vi "Stress Control Test.vi"() -> ()   [LabVIEW 2014]
uses:
  support/Instrument Status.ctl
  Spectrometer/Laser.ctl
  Spectrometer/Spectrometer Config.ctl
  Spectrometer/Laser Settings.ctl
  Spectrometer/Filter.ctl
  Spectrometer/Grating Detector Settings.ctl
  Spectrometer/Grating.ctl
  Spectrometer/Detector.ctl
  Spectrometer/Acquisition Settings.ctl
  Switches and Mirrors/SwitchesMirrors Config.ctl
  Switches and Mirrors/SwitchesMirrors Status.ctl
  Camera/Camera Config.ctl
  Camera/Camera Settings.ctl
  StressControl Config.ctl
  StressControl Refnums.ctl
  Parameter Analyzer/Parameter Analyzer Config.ctl
  Parameter Analyzer/Parameter Analyzer Integration Parameters.ctl
  Parameter Analyzer/Parameter Analyzer SMU Sweeping.ctl
  Parameter Analyzer/Parameter Analyzer Sweep Spacing.ctl
  Parameter Analyzer/Parameter Analyzer SMU Range.ctl
  Parameter Analyzer/Parameter Analyzer SMU Sampling.ctl
  Parameter Analyzer/Parameter Analyzer Sampling Parameters.ctl
  Parameter Analyzer/Parameter Analyzer Stop Sampling Conditions.ctl
  Switching Matrix/Switching Matrix Config.ctl
  XYZ Stage/XYZ Config.ctl
  XYZ Stage/XYZ Connection Settings.ctl
  XYZ Stage/XYZ Stage Control.ctl
  XYZ Stage/XYZ Coordinate Control.ctl
  Autofocus/AutoFocus Config.ctl
  Autofocus/ZScan.ctl
  <vilib>/Analysis/Matrix/Datatypes/RealMatrix.ctl
  Measurements/Strain Measurement/Strain Measurement Config.ctl
  Measurements/Plot Data/PlotData Config.ctl
  Measurements/Plot Data/Measurement.ctl
  Measurements/Plot Data/WhichInstrument.ctl
  Parameter Analyzer/Electrical Data.ctl
  Spectrometer/Spectral Data.ctl
  Measurements/Instrument Sequence/Instrument Steps.ctl
  Measurements/Instrument Sequence/Action.ctl
  Measurements/Instrument Sequence/Instrument List.ctl
  support/User Event - Stop/User Event - Stop.lvlib
  support/Message Queue/Message Queue.lvlib
  <vilib>/Analysis/Matrix/NI_Matrix.lvlib
panel:
  out "Instrument Status":T1
  in  "Mechanism Motion":u16(ring) items=["Absolute", "Relative"]
  in  "Apply Stress":bool
  out "Position (°)":dbl format="%.6g"
  in  "Destination (°)":dbl min=-2000000000.0 max=2000000000.0 format="%.6f"
  in  "Stop":bool
  out "Last Operation":string
  in  "Exit":bool
  # "LICENSED MATERIALS – PROPERTY OF IBM\nCopyright IBM Corp. 2016,\nALL RIGHTS RESERVED"
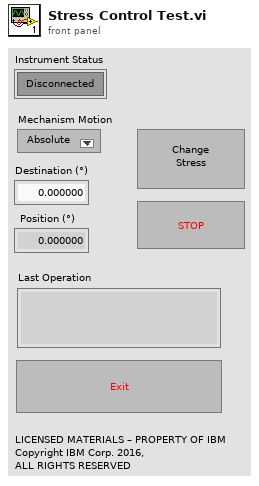
[diagram p1: front panel]
types:
  T1 = typedef "Instrument Status.ctl" = bool
  T2 = typedef "Message Queue.lvlib/All Message Queues.ctl" = cluster{"Message Handler Loop":refnum<queue>, "Parameter Analyzer":refnum<queue>, "Switching Matrix":refnum<queue>, "Stress Control":refnum<queue>, "Optical Spectrometer":refnum<queue>, "Switches & Mirrors":refnum<queue>, "Camera":refnum<queue>, "XYZ Stage":refnum<queue>, "AutoFocus":refnum<queue>, "Optoelectronic":refnum<queue>, "Save Data":refnum<queue>, "Plot Data":refnum<queue>, "Instrument Sequence":refnum<queue>, "Strain Measurement":refnum<queue>}
  T3 = typedef "Notifiers.ctl" = cluster{"Message Handler Loop":T4, "Parameter Analyzer":T5, "Switching Matrix":T6, "Stress Control":T7, "Optical Spectrometer":T8, "Switches & Mirrors":T9, "Camera":T10, "XYZ Stage":T11, "AutoFocus":T12, "Optoelectronic":T13, "Save Data":T14, "Plot Data":T14, "Instrument Sequence":T15, "Strain Measurement":cluster{"Status":refnum<notifier>, "Exit":refnum<notifier>, "Ready":refnum<notifier>}}
  T4 = typedef "Message Handler Loop Notifiers.ctl" = cluster{"Status":refnum<notifier>, "Instrument Data":refnum<notifier>, "Exit":refnum<notifier>, "Ready":refnum<notifier>}
  T5 = typedef "Parameter Analyzer Notifiers.ctl" = cluster{"Status":refnum<notifier>, "Instrument Data":refnum<notifier>, "Measurement":refnum<notifier>, "Exit":refnum<notifier>, "Ready":refnum<notifier>}
  T6 = typedef "Switching Matrix Notifiers.ctl" = cluster{"Status":refnum<notifier>, "Instrument Data":refnum<notifier>, "Measurement":refnum<notifier>, "Exit":refnum<notifier>, "Ready":refnum<notifier>}
  T7 = typedef "StressControl Notifiers.ctl" = cluster{"Status":refnum<notifier>, "Instrument Data":refnum<notifier>, "Measurement":refnum<notifier>, "Exit":refnum<notifier>, "Ready":refnum<notifier>}
  T8 = typedef "Spectrometer Notifiers.ctl" = cluster{"Status":refnum<notifier>, "Instrument Data":refnum<notifier>, "Measurement":refnum<notifier>, "Exit":refnum<notifier>, "Ready":refnum<notifier>}
  T9 = typedef "SwitchesMirrors Notifiers.ctl" = cluster{"Status":refnum<notifier>, "Instrument Data":refnum<notifier>, "Exit":refnum<notifier>, "Ready":refnum<notifier>}
  T10 = typedef "Camera Notifiers.ctl" = cluster{"Status":refnum<notifier>, "Instrument Data":refnum<notifier>, "Measurement":refnum<notifier>, "Exit":refnum<notifier>, "Ready":refnum<notifier>}
  T11 = typedef "XYZ Notifications.ctl" = cluster{"Status":refnum<notifier>, "Instrument Data":refnum<notifier>, "Measurement":refnum<notifier>, "Exit":refnum<notifier>, "Ready":refnum<notifier>}
  T12 = typedef "Autofocus Notifiers.ctl" = cluster{"Status":refnum<notifier>, "Instrument Data":refnum<notifier>, "Measurement":refnum<notifier>, "Exit":refnum<notifier>, "Ready":refnum<notifier>}
  T13 = typedef "Optoelectronic Notifiers.ctl" = cluster{"Status":refnum<notifier>, "Instrument Data":refnum<notifier>, "Measurement":refnum<notifier>, "Exit":refnum<notifier>, "Ready":refnum<notifier>}
  T14 = typedef "SaveData Notifiers.ctl" = cluster{"Status":refnum<notifier>, "Exit":refnum<notifier>, "Ready":refnum<notifier>}
  T15 = typedef "Instrument Sequence Notifiers.ctl" = cluster{"Status":refnum<notifier>, "Instrument Data":refnum<notifier>, "Measurement":refnum<notifier>, "Exit":refnum<notifier>, "Ready":refnum<notifier>}
  T16 = typedef "Configuration.ctl" = cluster{"Parameter Analizer":T17, "Switching Matrix":T25, "Stress Control":T26, "Optical Spectrometer":T27, "Switches & Mirrors":T35, "Camera":T37, "XYZ Stage":T39, "AutoFocus":T43, "Sava Data":T46, "PlotData":T51, "Instrument Sequence":T57, "Strain Measurement":T58}
  T17 = typedef "Parameter Analyzer Config.ctl" = cluster{"Parameter Analyzer VISA Session":refnum<visa-resource-name>, "Sweeping Time Parameters":T18, "Acquisition Mode":enum32{"Sweeping Mode", "Sampling Mode"}, "Status Polling Time (ms)":u32, "Comment":string, "SMU 1 - Sweeping":T19, "SMU 2 - Sweeping":T19, "SMU 3 - Sweeping":T19, "SMU 4 - Sweeping":T19, "Sweep Spacing":T20, "Range":T21, "SMU1 - Sampling":T22, "SMU2 - Sampling":T22, "SMU3 - Sampling":T22, "SMU4 - Sampling":T22, "Sampling Time Parameters":T23, "Stop Condition":T24}
  T18 = typedef "Parameter Analyzer Integration Parameters.ctl" = cluster{"Integration Time":u32, "Short Integration Time (s)":dbl, "Long Integration Time (s)":dbl, "Wait Time Parameter":dbl}
  T19 = typedef "Parameter Analyzer SMU Sweeping.ctl" = cluster{"Start / Offset":dbl, "Stop / Ratio":dbl, "Step \n(linear only)":dbl, "Compliance":dbl, "Power \nCompliance":dbl, "Mode":u32, "Function":i32, "Sweep Mode":bool}
  T20 = typedef "Parameter Analyzer Sweep Spacing.ctl" = u16
  T21 = typedef "Parameter Analyzer SMU Range.ctl" = u16
  T22 = typedef "Parameter Analyzer SMU Sampling.ctl" = cluster{"Source":dbl, "Compliance":dbl, "Mode":u32, "Function":bool}
  T23 = typedef "Parameter Analyzer Sampling Parameters.ctl" = cluster{"Initial Interval (s)":dbl, "Number of Samples":i32, "Total Sampling Time (s)":dbl, "Hold Time (s)":dbl, "Sampling Mode":i32, "Sampling Time":i32}
  T24 = typedef "Parameter Analyzer Stop Sampling Conditions.ctl" = cluster{"Enable Delay (s)":dbl, "Name":string, "Threshold":dbl, "num. of events":i32, "Event":i32, "Stop Condition Enable":bool}
  T25 = typedef "Switching Matrix Config.ctl" = cluster{"Switching Matrix VISA Session":refnum<visa-resource-name>, "Connections":cluster{"Connections":bool[], "Connection Type":enum16{"Disconnected", "Make - Break", "Break - Make"}}[]}
  T26 = typedef "StressControl Config.ctl" = cluster{"Stress Control VISA Session":refnum<visa-resource-name>, "Axis":i32, "Motion":u16, "Destination (°)":dbl, "Speed (°/s)":dbl, "Position (°)":dbl}
  T27 = typedef "Spectrometer Config.ctl" = cluster{"Laser Settings":T28, "Spectrometer Settings":T31, "Acquisition Settings":T34, "Path":path}
  T28 = typedef "Laser Settings.ctl" = cluster{"Laser Wavelength":T29, "Neutral Density Filter":T30}
  T29 = typedef "Laser.ctl" = enum16{"633 nm", "784 nm", "532 nm", "365 nm"}
  T30 = typedef "Filter.ctl" = enum16{"100%", "50%", "25%", "10%", "1%", "0.1%", "0.01%"}
  T31 = typedef "Grating Detector Settings.ctl" = cluster{"Confocal Hole Size (µm)":dbl, "Grating":T32, "Detector":T33}
  T32 = typedef "Grating.ctl" = u16
  T33 = typedef "Detector.ctl" = enum16{"InGaAs Array", "Silicon CCD"}
  T34 = typedef "Acquisition Settings.ctl" = cluster{"Acquisition Mode":enum16{"Single Window", "Multi-Window"}, "Spectal Position (nm)":dbl, "From (nm)":dbl, "To (nm)":dbl, "Integration Time (s)":dbl, "Number of Accumulations":i32, "AutoScanning":bool, "Spike Removal":bool}
  T35 = typedef "SwitchesMirrors Config.ctl" = cluster{"Relay VISA Session":refnum<visa-resource-name>, "Switches":T36, "Delays (ms)":cluster{"Laser":u32, "Video":u32}}
  T36 = typedef "SwitchesMirrors Status.ctl" = cluster{"Laser":bool, "Video":bool}
  T37 = typedef "Camera Config.ctl" = cluster{"Settings":T38}
  T38 = typedef "Camera Settings.ctl" = cluster{"Pixel clock":i32, "Frame rate":dbl, "Exposure time":dbl, "Master Gain":i32, "Red Gain":i32, "Green Gain":i32, "Blue Gain":i32, "Auto Gain":bool, "White-balance":bool, "Color Correction":bool}
  T39 = typedef "XYZ Config.ctl" = cluster{"Connection Settings":T40, "Manual Control":T41, "Coordinate Control":T42}
  T40 = typedef "XYZ Connection Settings.ctl" = cluster{"Tango VISA":refnum<visa-resource-name>, "Baudrate":i32, "Show Protocol?":bool}
  T41 = typedef "XYZ Stage Control.ctl" = cluster{"North":bool, "South":bool, "West":bool, "East":bool, "Up":bool, "Down":bool, "Stop":bool, "XY Step":dbl, "Z step":dbl}
  T42 = typedef "XYZ Coordinate Control.ctl" = cluster{"Motion Mode":enum16{"Absolute", "Relative"}, "Destination [mm]":dbl[]}
  T43 = typedef "AutoFocus Config.ctl" = cluster{"Matching Criteria":cluster{"Minimum Score":sgl, "Color Score Weight":sgl, "Minimum Contrast":i32, "Match Mode":u32, "Match Feature Mode":u32, "Subpixel Accuracy":bool, "Color Sensitivity":u32, "Search Strategy":u32}, "Z Scan Parameters":T44, "Displacement":dbl, "Transformation Matrix":T45}
  T44 = typedef "ZScan.ctl" = cluster{"Z Range":ext, "Resolution":dbl, "Initial Direction":enum16{"Up", "Down"}, "Focus Threshold":dbl, "Ascent Constant":dbl}
  T45 = typedef "NI_Matrix.lvlib/RealMatrix.ctl" = dbl[][]
  T46 = typedef "SaveData Config.ctl" = cluster{"Workspace Info":T47, "Instrument Configuration":T48, "Stress Motor Position":dbl, "Electrical Measurement":cluster{"Sequence":dbl[], "V1":dbl[], "V2":dbl[], "V3":dbl[], "V4":dbl[], "I1":dbl[], "I2":dbl[], "I3":dbl[], "I4":dbl[]}, "Optical Spectrum":T50}
  T47 = typedef "SaveData Workspace Info.ctl" = cluster{"Device Name":string, "Device Info":string, "Path":path}
  T48 = typedef "SaveData Instrument Configuration.ctl" = cluster{"Instrument":T49, "Configuration":string}
  T49 = typedef "Instrument List.ctl" = enum32{"Unknown Instrument", "Switching Matrix", "Parameter Analyzer", "Optical Spectrometer", "Optoelectronic", "Autofocus"}
  T50 = typedef "Spectral Data.ctl" = cluster{"Intensity":dbl[], "Wavelength":dbl[], "Energy":dbl[], "Raman Shift":dbl[], "Detector Temperature":dbl}
  T51 = typedef "PlotData Config.ctl" = cluster{"Sliders":cluster{"Strain Sequence":i32, "Instrument Sequence":i32}, "Measurement":T52, "Instrument Steps":T55, "Strain Points":dbl[]}
  T52 = typedef "Measurement.ctl" = cluster{"Which Instrument?":T53, "Electrical Measurement":T54, "Measurement Mode":enum16{"Sweeping Mode", "Sampling Mode"}, "Optical Spectrum":T50}
  T53 = typedef "WhichInstrument.ctl" = enum16{"No Plot", "Spectrometer", "Parameter Analyzer", "Optoelectronic"}
  T54 = typedef "Electrical Data.ctl" = cluster{"Sequence":dbl[], "V1":dbl[], "V2":dbl[], "V3":dbl[], "V4":dbl[], "I1":dbl[], "I2":dbl[], "I3":dbl[], "I4":dbl[]}
  T55 = typedef "Instrument Steps.ctl" = cluster{"Action":T56, "Configuration":variant, "Instrument":T49, "Status":enum8{"False", "True", "Mixed"}}[]
  T56 = typedef "Action.ctl" = enum32{"Configure", "Measure"}
  T57 = typedef "Instrument Sequence Config.ctl" = cluster{"Caller VI":enum16{"User", "Stress Measurement VI"}}
  T58 = typedef "Strain Measurement Config.ctl" = cluster{"Stress Sequence ":cluster{"Max Motor Position":ext, "# Intermediate Points":u32, "Initial Direction":enum16{"Tension", "Compression"}}, "Track?":bool}
  T59 = typedef "StressControl Refnums.ctl" = cluster{"Instrument Status":refnum<vi>, "Position":refnum<vi>, "Mecahnism Motion":refnum<vi>, "Destination":refnum<vi>, "Apply Stress":refnum<vi>, "Stop":refnum<vi>, "Stress Control VISA":refnum<vi>}
  T60 = cluster{"SMU 1 - Sweeping":cluster{"Start / Offset":dbl, "Stop / Ratio":dbl, "Step (linear only)":dbl, "Compliance":dbl, "Power Compliance":dbl, "Mode":u32, "Function":i32, "Sweep Mode":bool}, "SMU 2 - Sweeping":cluster{"Start / Offset":dbl, "Stop / Ratio":dbl, "Step (linear only)":dbl, "Compliance":dbl, "Power Compliance":dbl, "Mode":u32, "Function":i32, "Sweep Mode":bool}, "SMU 3 - Sweeping":cluster{"Start / Offset":dbl, "Stop / Ratio":dbl, "Step (linear only)":dbl, "Compliance":dbl, "Power Compliance":dbl, "Mode":u32, "Function":i32, "Sweep Mode":bool}, "SMU 4 - Sweeping":cluster{"Start / Offset":dbl, "Stop / Ratio":dbl, "Step (linear only)":dbl, "Compliance":dbl, "Power Compliance":dbl, "Mode":u32, "Function":i32, "Sweep Mode":bool}, "Sweep Spacing":u16, "Range":u16}
  T61 = cluster{"SMU1 - Sampling":cluster{"Source":dbl, "Compliance":dbl, "Mode":u32, "Function":bool}, "SMU2 - Sampling":cluster{"Source":dbl, "Compliance":dbl, "Mode":u32, "Function":bool}, "SMU3 - Sampling":cluster{"Source":dbl, "Compliance":dbl, "Mode":u32, "Function":bool}, "SMU4 - Sampling":cluster{"Source":dbl, "Compliance":dbl, "Mode":u32, "Function":bool}, "Sampling Parameters":cluster{"Initial Interval (s)":dbl, "Number of Samples":i32, "Total Sampling Time (s)":dbl, "Hold Time (s)":dbl, "Sampling Mode":i32, "Sampling Time":i32}, "Stop Condition":cluster{"Enable Delay (s)":dbl, "Name":string, "Threshold":dbl, "num. of events":i32, "Event":i32, "Stop Condition Enable":bool}}
  T62 = cluster{"PlotData - Instrument Sequence":i32, "PlotData - Strain Sequence":i32}
  T63 = cluster{"Start / Offset":dbl, "Stop / Ratio":dbl, "Step (linear only)":dbl, "Compliance":dbl, "Power Compliance":dbl, "Mode":u32, "Function":i32, "Sweep Mode":bool}
  T64 = cluster{"Source":dbl, "Compliance":dbl, "Mode":u32, "Function":bool}
  T65 = cluster{"Initial Interval (s)":dbl, "Number of Samples":i32, "Total Sampling Time (s)":dbl, "Hold Time (s)":dbl, "Sampling Mode":i32, "Sampling Time":i32}
  T66 = cluster{"Enable Delay (s)":dbl, "Name":string, "Threshold":dbl, "num. of events":i32, "Event":i32, "Stop Condition Enable":bool}
  T67 = cluster{"Connections":bool[], "Connection Type":enum16{"Disconnected", "Make - Break", "Break - Make"}}[]
  T68 = cluster{"Minimum Score":sgl, "Color Score Weight":sgl, "Minimum Contrast":i32, "Match Mode":u32, "Match Feature Mode":u32, "Subpixel Accuracy":bool, "Color Sensitivity":u32, "Search Strategy":u32}
  T69 = cluster{"Max Motor Position":ext, "# Intermediate Points":u32, "Initial Direction":enum16{"Tension", "Compression"}}
  T70 = enum32{"invalid app kind", "Development System", "Run Time System", "Student Edition", "Embedded LabVIEW", "Evaluation", "Custom"}
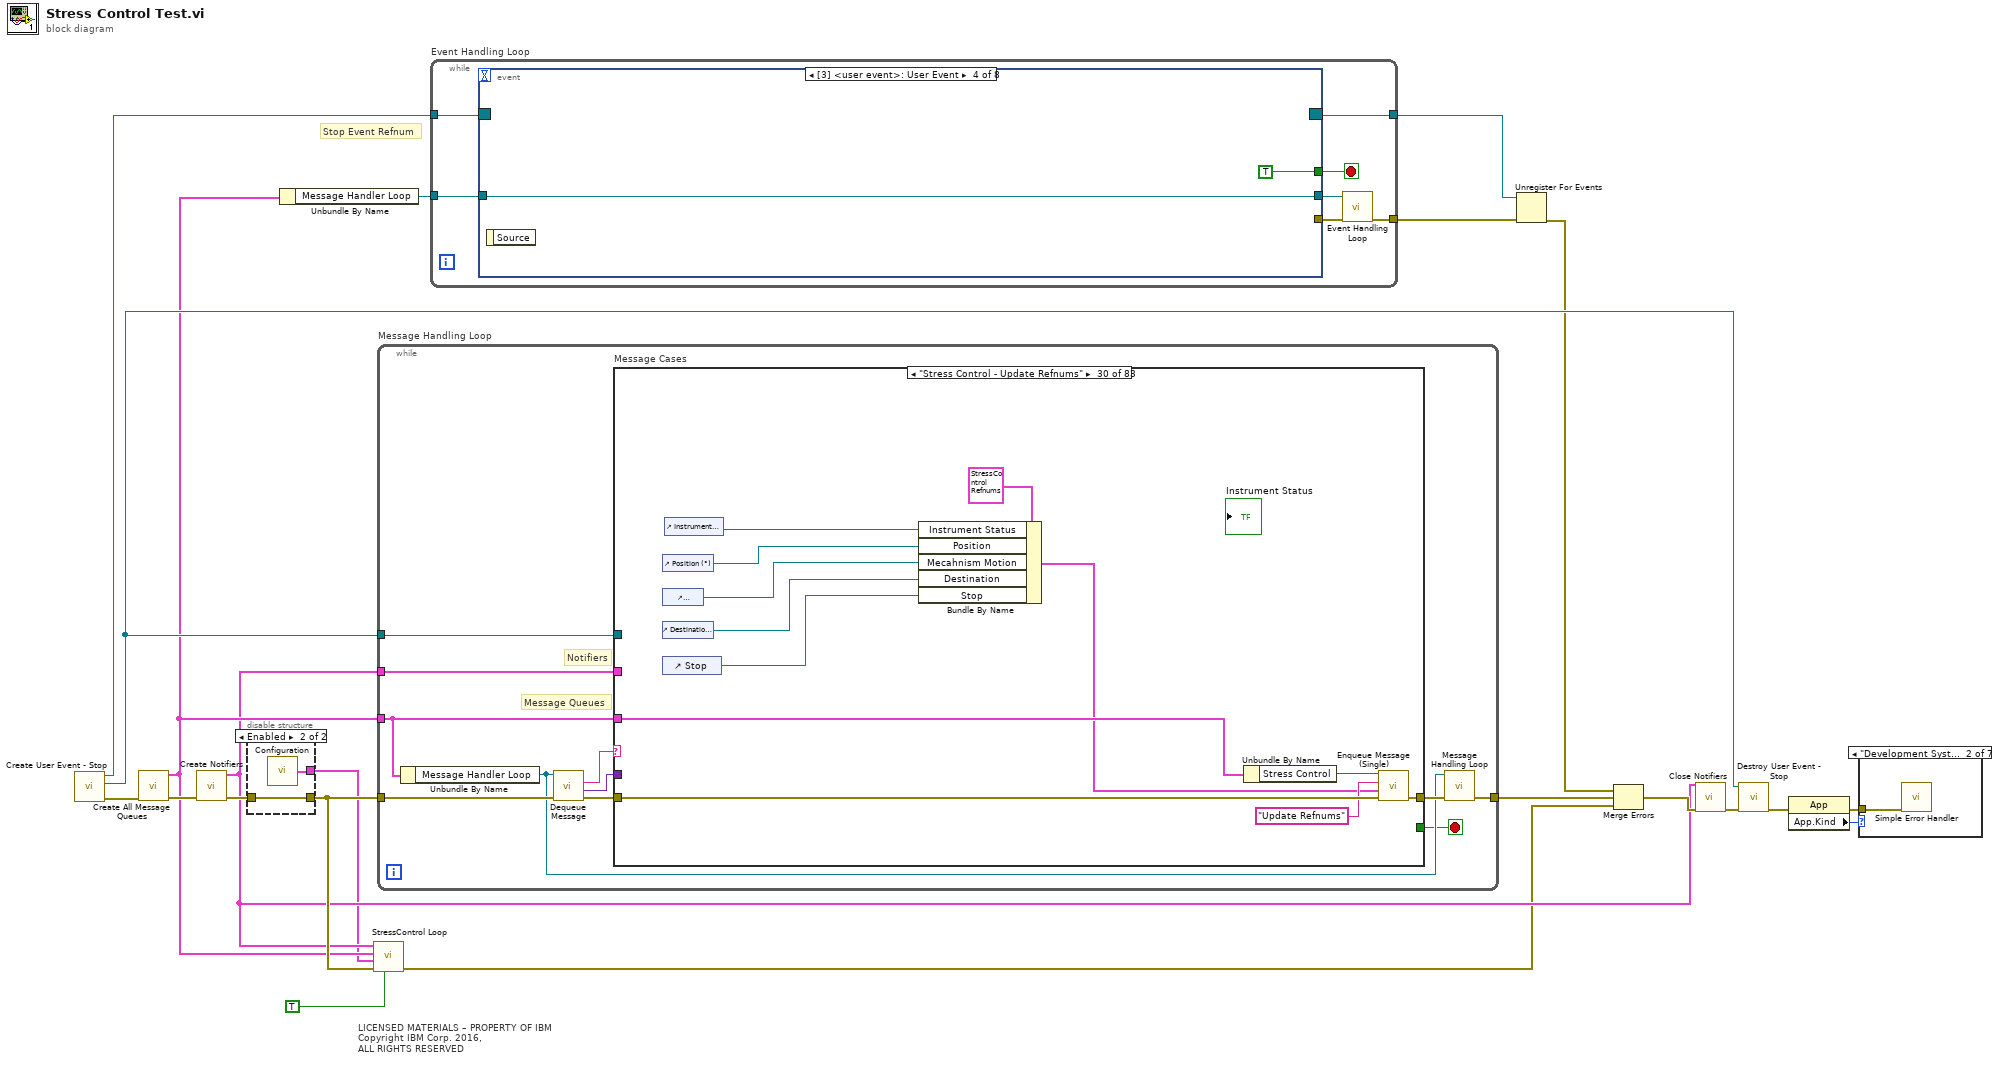
[diagram p0: block diagram]
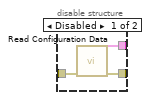
[diagram p2: hidden frame]
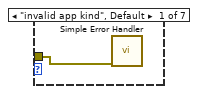
[diagram p3: hidden frame]
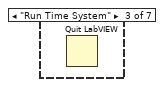
[diagram p4: hidden frame]
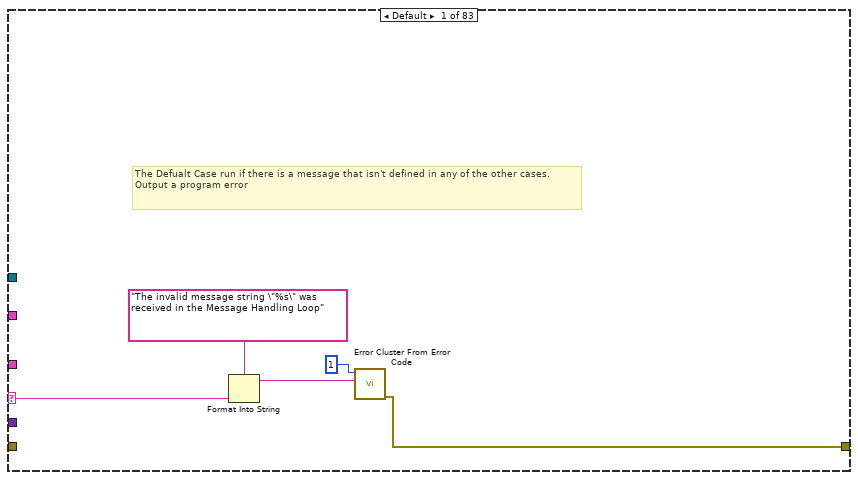
[diagram p9: hidden frame]
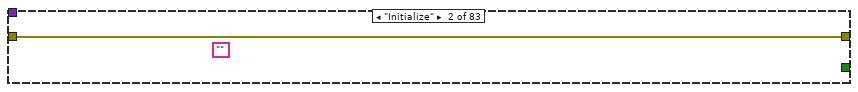
[diagram p10: hidden frame]
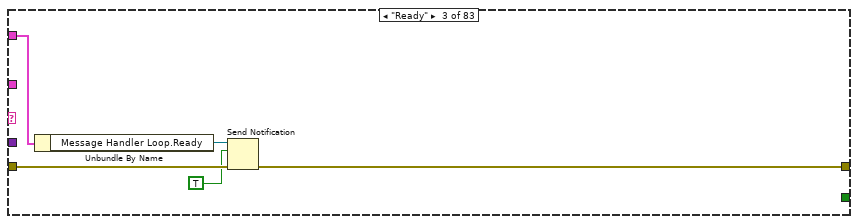
[diagram p11: hidden frame]
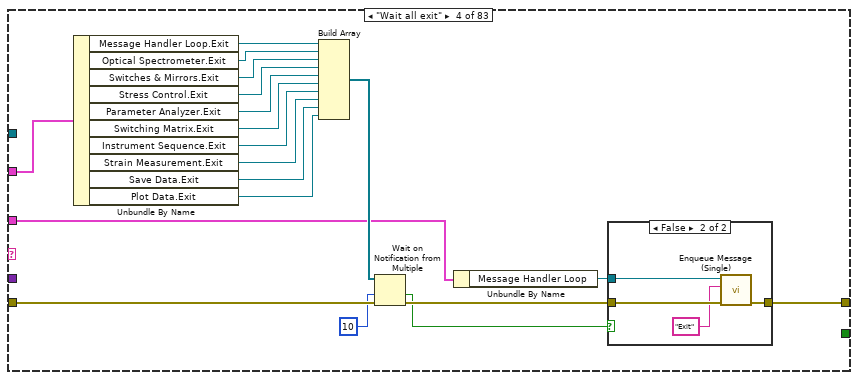
[diagram p12: hidden frame]
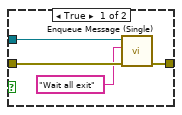
[diagram p13: hidden frame]
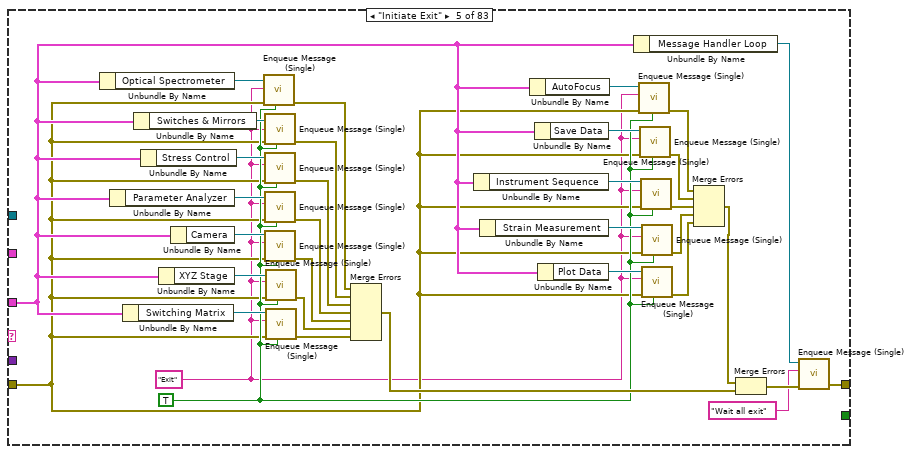
[diagram p14: hidden frame]
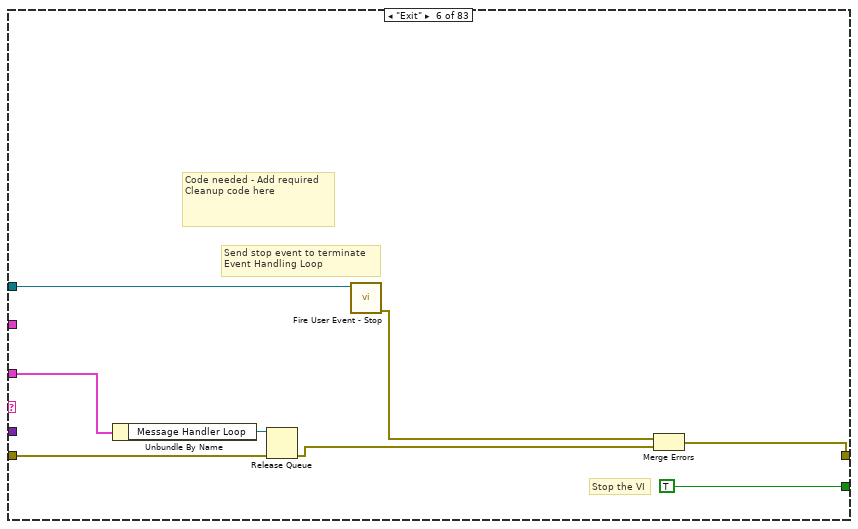
[diagram p15: hidden frame]
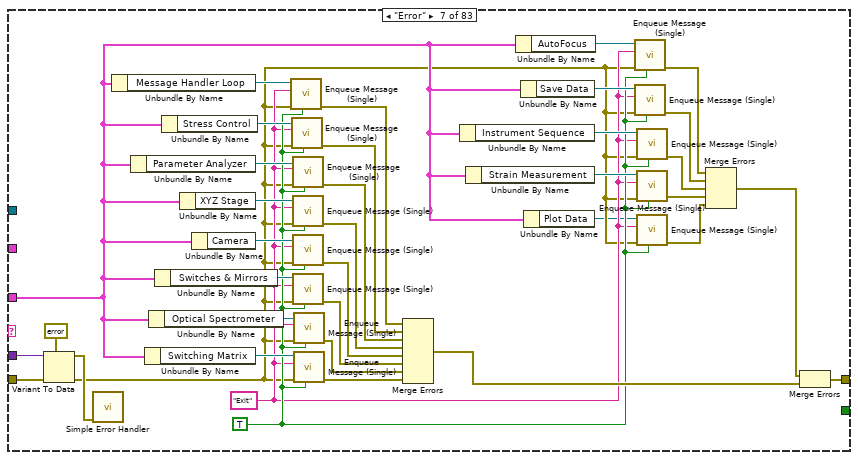
[diagram p16: hidden frame]
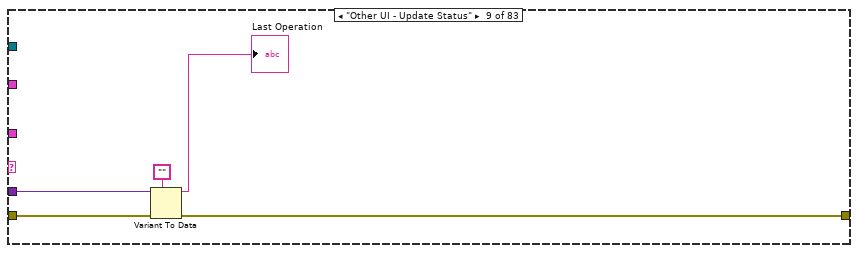
[diagram p18: hidden frame]
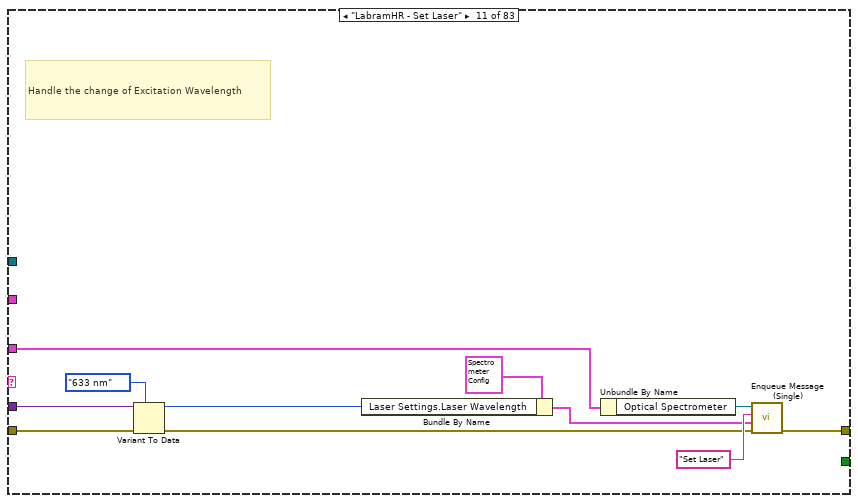
[diagram p20: hidden frame]
diagram:
  # "LICENSED MATERIALS – PROPERTY OF IBM\nCopyright IBM Corp. 2016,\nALL RIGHTS RESERVED"
  # "Stop Event Refnum"
  n1 = call "Create User Event - Stop.vi"() -> ("error out"=w11:errorcluster, "User Event - Stop"=w14:refnum<user-event>, "Stop Event Registration Refnum"=w21:refnum<event-registration>)  [unwired: 1 in, 8 out]
  n2 = call "Create All Message Queues.vi"("error in (no error)"=w11) -> ("error out"=w10:errorcluster, "Message Queues out"=w7:T2)  [unwired: 9 out]
  n3 = call "Create Notifiers.vi"("error in"=w10) -> ("error out"=w9:errorcluster, "Notifiers"=w6:T3)  [unwired: 9 out]
  n4 = disable-structure shown="Enabled" {
    disable-tunnel: w9 -> [w24 w26]
    disable-tunnel: [w23 w26] -> w8
    disable-tunnel: [w22 w25] -> w2
    frame Disabled {
      n5 = call "Read Configuration Data.vi"("error in"=w24) -> ("error out"=w23:errorcluster, "System Configuration"=w22:T16)  [unwired: 9 out]
    }
    frame Enabled {
      n6 = call "Configuration.vi"() -> ("IBM OptoElectroMechanics Configuration"=w25:T16)
    }
  }
  n7 = Unbundle By Name(w7) -> ("Message Handler Loop"=w19:refnum<queue>)
  n8 = call "StressControl Loop.vi"("Used functions"=TRUE, "error in"=w8, "IBM OptoElectroMechanics Configuration"=w2, "Message Queues out"=w7, "Notifiers"=w6) -> ("error out"=w3:errorcluster)  [unwired: 6 out]
  n9 = while "Message Handling Loop" {
    tunnel: w8 -> [w37]
    tunnel: [w34] -> w4
    tunnel: w7 -> [w28]
    tunnel: w14 -> [w30]
    tunnel: w6 -> [w27]
    stop <- w29 stop-if-true
    # "Notifiers"
    # "Message Queues"
    n10 = Unbundle By Name(w28) -> ("Message Handler Loop"=w33:refnum<queue>)
    n11 = call "Dequeue Message.vi"("error in (no error)"=w37, "Message Queue"=w33) -> ("error out"=w36:errorcluster, "Message Data"=w31:variant, "Message"=w32:string)  [unwired: 7 out]
    n12 = case "Message Cases" shown="\"Stress Control - Update Refnums\"" w32 {
      selector: w32 -> [w42 _ _ _ _ _ _ _ _ _ _ _ _ _ _ _ _ _ _ _ _ _ _ _ _ _ _ _ _ _ _ _ _ _ _ _ _ _ _ _ _ _ _ _ _ _ _ _ _ _ _ _ _ _ _ _ _ _ _ _ _ _ _ _ _ _ _ _ _ _ _ _ _ _ _ _ _ _ _ _ _ _ _]
      tunnel: w36 -> [_ w43 w47 w66 w79 w116 w143 w155 w160 w161 w168 w183 w194 w205 w216 w227 w238 w242 w247 w249 w257 w270 w281 w283 w293 w295 w300 w305 w311 w322 w336 w347 w358 w369 w370 w375 w386 w397 w414 w431 w432 w437 w445 w456 w460 w465 w470 w481 w492 w493 w504 w515 w526 w527 w532 w537 w542 w547 w552 w557 w562 w567 w570 w575 w580 w585 w590 w593 w598 w603 w608 w619 w624 w629 w634 w637 w642 w647 w652 w657 w660 w673 w674]
      tunnel: [w38 w43 w48 w55 w95 w117 w152 w155 w157 w161 w166 w179 w190 w202 w213 w223 w236 w239 w244 w249 w260 w269 w280 w283 w292 w299 w304 w305 w310 w321 w335 w346 w357 w368 w374 w375 w380 w392 w403 w423 w434 w437 w448 w459 w464 w469 w470 w476 w488 w493 w499 w510 w521 w530 w535 w540 w545 w550 w555 w560 w565 w567 w569 w574 w579 w584 w589 w595 w600 w605 w608 w616 w623 w628 w633 w636 w641 w646 w651 w656 w660 w668 w674] -> w35
      tunnel: w31 -> [_ _ _ _ _ _ w154 _ w159 _ w172 w182 w193 w204 w215 w226 w237 _ _ _ w253 w271 w282 _ w294 _ _ _ w309 _ w329 w341 w352 w363 _ _ w385 w396 w413 w430 _ _ w442 w453 _ _ _ w480 w491 _ w503 w514 w525 _ _ _ _ _ _ _ _ _ _ _ _ _ _ _ _ _ _ w618 _ _ _ _ _ _ _ _ _ w672 _]
      tunnel: w30 -> [_ _ _ _ _ w114 _ _ _ _ _ _ _ _ _ _ _ _ _ _ _ _ _ _ _ _ _ _ _ _ _ _ _ _ _ _ _ _ _ _ _ _ _ _ _ _ _ _ _ _ _ _ _ _ _ _ _ _ _ _ _ _ _ _ _ _ _ _ _ _ _ _ _ _ _ _ _ _ _ _ _ _ _]
      tunnel: [_ _ _ _ _ TRUE _ _ _ _ _ _ _ _ _ _ _ _ _ _ _ _ _ _ _ _ _ _ _ _ _ _ _ _ _ _ _ _ _ _ _ _ _ _ _ _ _ _ _ _ _ _ _ _ _ _ _ _ _ _ _ _ _ _ _ _ _ _ _ _ _ _ _ _ _ _ _ _ _ _ _ _ _] -> w29
      tunnel: w28 -> [_ _ _ w54 w82 w111 w124 _ _ _ w171 w178 w187 w200 w211 w220 w232 w240 w245 _ w258 w266 w277 _ w290 w297 w302 _ _ w318 w332 w343 w354 w365 w372 _ w382 w391 w402 w422 w433 _ w446 w457 w462 w467 _ w475 w487 _ w498 w509 w520 w529 w534 w539 w544 w549 w554 w559 w564 _ w572 w577 w582 w587 w592 w597 w602 w607 _ w613 w620 w625 w630 w639 w644 w649 w654 w659 _ w667 _]
      tunnel: w27 -> [_ _ w46 w67 _ _ _ _ _ _ _ _ _ _ _ _ _ _ _ _ _ _ _ _ _ _ _ _ _ _ _ _ _ _ _ _ _ _ _ _ _ _ _ _ _ _ _ _ _ _ _ _ _ _ _ _ _ _ _ _ _ _ _ _ _ _ _ _ _ _ _ _ _ _ _ _ _ _ _ _ _ _ _]
      frame Default {
        # "The Defualt Case run if there is a message that isn't defined in any of the other cases.\nOutput a program error"
        n13 = Format Into String(format string="The invalid message string \"%s\" was  received in the Message Handling Loop", w42) -> (resulting string=w40:string)  [unwired: 2 in, 1 out]
        n14 = call <vilib>:"Error Cluster From Error Code.vi"("error message (\"\")"=w40, "error code (0)"=1) -> ("error out"=w38:errorcluster)  [unwired: 2 in, 5 out]
      }
      frame "Initialize" {
        (unwired) ""
      }
      frame "Ready" {
        n15 = Unbundle By Name(w46) -> ("Message Handler Loop.Ready"=w45:refnum<notifier>)
        n16 = Send Notification(notification=TRUE, notifier=w45, error in (no error)=w47) -> (error out=w48:errorcluster)  [unwired: 1 out]
      }
      frame "Wait all exit" {
        n17 = Unbundle By Name(w67) -> ("Message Handler Loop.Exit"=w64:refnum<notifier>, "Optical Spectrometer.Exit"=w63:refnum<notifier>, "Switches & Mirrors.Exit"=w62:refnum<notifier>, "Stress Control.Exit"=w61:refnum<notifier>, "Parameter Analyzer.Exit"=w60:refnum<notifier>, "Switching Matrix.Exit"=w59:refnum<notifier>, "Instrument Sequence.Exit"=w52:refnum<notifier>, "Strain Measurement.Exit"=w51:refnum<notifier>, "Save Data.Exit"=w50:refnum<notifier>, "Plot Data.Exit"=w49:refnum<notifier>)
        n18 = Build Array(w64, w63, w62, w61, w60, w59, w52, w51, w50, w49) -> (w58:refnum<notifier>[])
        n19 = Wait on Notification from Multiple(0:w58, 2:10 ("timeout in ms (-1)"), 3:w66) -> (10:w53:bool, 11:w56:errorcluster)  [unwired: 3 out]
        n20 = Unbundle By Name(w54) -> ("Message Handler Loop"=w57:refnum<queue>)
        n21 = case shown="False" w53 {
          tunnel: w57 -> [w71 w75]
          tunnel: w56 -> [w70 w74]
          tunnel: [w69 w73] -> w55
          frame True {
            n22 = call "Enqueue Message (Single).vi"("error in (no error)"=w70, "Message"="Wait all exit", "Message Queue"=w71) -> ("error out"=w69:errorcluster)  [unwired: 1 in, 7 out]
          }
          frame False {
            n23 = call "Enqueue Message (Single).vi"("error in (no error)"=w74, "Message"="Exit", "Message Queue"=w75) -> ("error out"=w73:errorcluster)  [unwired: 1 in, 7 out]
          }
        }
      }
      frame "Initiate Exit" {
        w80 = TRUE ("Priority Message? (F)")
        w77 = "Exit" ("Message")
        n24 = Unbundle By Name(w82) -> ("Optical Spectrometer"=w99:refnum<queue>)
        n25 = Unbundle By Name(w82) -> ("Parameter Analyzer"=w96:refnum<queue>)
        n26 = Unbundle By Name(w82) -> ("Switching Matrix"=w91:refnum<queue>)
        n27 = Unbundle By Name(w82) -> ("Switches & Mirrors"=w98:refnum<queue>)
        n28 = Unbundle By Name(w82) -> ("Stress Control"=w97:refnum<queue>)
        n29 = Unbundle By Name(w82) -> ("XYZ Stage"=w109:refnum<queue>)
        n30 = Unbundle By Name(w82) -> ("Camera"=w100:refnum<queue>)
        n31 = call "Enqueue Message (Single).vi"("Priority Message? (F)"=w80, "error in (no error)"=w79, "Message"=w77, "Message Queue"=w99) -> ("error out"=w101:errorcluster)  [unwired: 1 in, 6 out]
        n32 = call "Enqueue Message (Single).vi"("Priority Message? (F)"=w80, "error in (no error)"=w79, "Message"=w77, "Message Queue"=w98) -> ("error out"=w102:errorcluster)  [unwired: 1 in, 6 out]
        n33 = call "Enqueue Message (Single).vi"("Priority Message? (F)"=w80, "error in (no error)"=w79, "Message"=w77, "Message Queue"=w97) -> ("error out"=w103:errorcluster)  [unwired: 1 in, 6 out]
        n34 = call "Enqueue Message (Single).vi"("Priority Message? (F)"=w80, "error in (no error)"=w79, "Message"=w77, "Message Queue"=w96) -> ("error out"=w104:errorcluster)  [unwired: 1 in, 6 out]
        n35 = call "Enqueue Message (Single).vi"("Priority Message? (F)"=w80, "error in (no error)"=w79, "Message"=w77, "Message Queue"=w100) -> ("error out"=w105:errorcluster)  [unwired: 1 in, 6 out]
        n36 = call "Enqueue Message (Single).vi"("Priority Message? (F)"=w80, "error in (no error)"=w79, "Message"=w77, "Message Queue"=w109) -> ("error out"=w106:errorcluster)  [unwired: 1 in, 6 out]
        n37 = call "Enqueue Message (Single).vi"("Priority Message? (F)"=w80, "error in (no error)"=w79, "Message"=w77, "Message Queue"=w91) -> ("error out"=w107:errorcluster)  [unwired: 1 in, 6 out]
        n38 = Merge Errors(w101, w102, w103, w104, w105, w106, w107) -> (w108:errorcluster)
        n39 = Unbundle By Name(w82) -> ("Instrument Sequence"=w88:refnum<queue>)
        n40 = Unbundle By Name(w82) -> ("Strain Measurement"=w84:refnum<queue>)
        n41 = Unbundle By Name(w82) -> ("AutoFocus"=w90:refnum<queue>)
        n42 = Unbundle By Name(w82) -> ("Save Data"=w89:refnum<queue>)
        n43 = Unbundle By Name(w82) -> ("Plot Data"=w81:refnum<queue>)
        n44 = Unbundle By Name(w82) -> ("Message Handler Loop"=w93:refnum<queue>)
        n45 = call "Enqueue Message (Single).vi"("Priority Message? (F)"=w80, "error in (no error)"=w79, "Message"=w77, "Message Queue"=w90) -> ("error out"=w87:errorcluster)  [unwired: 1 in, 6 out]
        n46 = call "Enqueue Message (Single).vi"("Priority Message? (F)"=w80, "error in (no error)"=w79, "Message"=w77, "Message Queue"=w89) -> ("error out"=w86:errorcluster)  [unwired: 1 in, 6 out]
        n47 = call "Enqueue Message (Single).vi"("Priority Message? (F)"=w80, "error in (no error)"=w79, "Message"=w77, "Message Queue"=w88) -> ("error out"=w85:errorcluster)  [unwired: 1 in, 6 out]
        n48 = call "Enqueue Message (Single).vi"("Priority Message? (F)"=w80, "error in (no error)"=w79, "Message"=w77, "Message Queue"=w84) -> ("error out"=w83:errorcluster)  [unwired: 1 in, 6 out]
        n49 = call "Enqueue Message (Single).vi"("Priority Message? (F)"=w80, "error in (no error)"=w79, "Message"=w77, "Message Queue"=w81) -> ("error out"=w78:errorcluster)  [unwired: 1 in, 6 out]
        n50 = Merge Errors(w87, w86, w85, w83, w78) -> (w76:errorcluster)
        n51 = Merge Errors(w76, w108) -> (w94:errorcluster)
        n52 = call "Enqueue Message (Single).vi"("error in (no error)"=w94, "Message"="Wait all exit", "Message Queue"=w93) -> ("error out"=w95:errorcluster)  [unwired: 1 in, 7 out]
      }
      frame "Exit" {
        # "Send stop event to terminate \nEvent Handling Loop"
        # "Stop the VI"
        # "Code needed - Add required Cleanup code here"
        n53 = Unbundle By Name(w111) -> ("Message Handler Loop"=w110:refnum<queue>)
        n54 = Release Queue(queue=w110, error in (no error)=w116) -> (error out=w115:errorcluster)  [unwired: 3 out]
        n55 = call "Fire User Event - Stop.vi"("User Event - Stop"=w114) -> ("error out"=w113:errorcluster)  [unwired: 1 in, 9 out]
        n56 = Merge Errors(w113, w115) -> (w117:errorcluster)
      }
      frame "Error" {
        w123 = TRUE ("Priority Message? (F)")
        w122 = "Exit" ("Message")
        n57 = Variant To Data(error in=w143, type=errorcluster {"status"=FALSE, "code"=0, "source"=""} ("error out"), Variant=w154) -> (data=w151:errorcluster, error out=w120:errorcluster)
        n58 = call <vilib>:"Simple Error Handler.vi"("error in (no error)"=w151) -> ()  [unwired: 1 in, 8 out]
        n59 = Unbundle By Name(w124) -> ("Message Handler Loop"=w134:refnum<queue>)
        n60 = Unbundle By Name(w124) -> ("Parameter Analyzer"=w149:refnum<queue>)
        n61 = Unbundle By Name(w124) -> ("Switching Matrix"=w144:refnum<queue>)
        n62 = Unbundle By Name(w124) -> ("Optical Spectrometer"=w145:refnum<queue>)
        n63 = Unbundle By Name(w124) -> ("Switches & Mirrors"=w135:refnum<queue>)
        n64 = Unbundle By Name(w124) -> ("Stress Control"=w148:refnum<queue>)
        n65 = Unbundle By Name(w124) -> ("XYZ Stage"=w150:refnum<queue>)
        n66 = Unbundle By Name(w124) -> ("Camera"=w136:refnum<queue>)
        n67 = call "Enqueue Message (Single).vi"("Priority Message? (F)"=w123, "error in (no error)"=w120, "Message"=w122, "Message Queue"=w134) -> ("error out"=w133:errorcluster)  [unwired: 1 in, 6 out]
        n68 = call "Enqueue Message (Single).vi"("Priority Message? (F)"=w123, "error in (no error)"=w120, "Message"=w122, "Message Queue"=w148) -> ("error out"=w142:errorcluster)  [unwired: 1 in, 6 out]
        n69 = call "Enqueue Message (Single).vi"("Priority Message? (F)"=w123, "error in (no error)"=w120, "Message"=w122, "Message Queue"=w149) -> ("error out"=w141:errorcluster)  [unwired: 1 in, 6 out]
        n70 = call "Enqueue Message (Single).vi"("Priority Message? (F)"=w123, "error in (no error)"=w120, "Message"=w122, "Message Queue"=w150) -> ("error out"=w140:errorcluster)  [unwired: 1 in, 6 out]
        n71 = call "Enqueue Message (Single).vi"("Priority Message? (F)"=w123, "error in (no error)"=w120, "Message"=w122, "Message Queue"=w136) -> ("error out"=w139:errorcluster)  [unwired: 1 in, 6 out]
        n72 = call "Enqueue Message (Single).vi"("Priority Message? (F)"=w123, "error in (no error)"=w120, "Message"=w122, "Message Queue"=w135) -> ("error out"=w138:errorcluster)  [unwired: 1 in, 6 out]
        n73 = call "Enqueue Message (Single).vi"("Priority Message? (F)"=w123, "error in (no error)"=w120, "Message"=w122, "Message Queue"=w145) -> ("error out"=w147:errorcluster)  [unwired: 1 in, 6 out]
        n74 = call "Enqueue Message (Single).vi"("Priority Message? (F)"=w123, "error in (no error)"=w120, "Message"=w122, "Message Queue"=w144) -> ("error out"=w146:errorcluster)  [unwired: 1 in, 6 out]
        n75 = Merge Errors(w133, w142, w141, w140, w139, w138, w147, w146) -> (w137:errorcluster)
        n76 = Unbundle By Name(w124) -> ("Instrument Sequence"=w130:refnum<queue>)
        n77 = Unbundle By Name(w124) -> ("Strain Measurement"=w126:refnum<queue>)
        n78 = Unbundle By Name(w124) -> ("AutoFocus"=w132:refnum<queue>)
        n79 = Unbundle By Name(w124) -> ("Save Data"=w131:refnum<queue>)
        n80 = Unbundle By Name(w124) -> ("Plot Data"=w119:refnum<queue>)
        n81 = call "Enqueue Message (Single).vi"("Priority Message? (F)"=w123, "error in (no error)"=w120, "Message"=w122, "Message Queue"=w132) -> ("error out"=w127:errorcluster)  [unwired: 1 in, 6 out]
        n82 = call "Enqueue Message (Single).vi"("Priority Message? (F)"=w123, "error in (no error)"=w120, "Message"=w122, "Message Queue"=w131) -> ("error out"=w128:errorcluster)  [unwired: 1 in, 6 out]
        n83 = call "Enqueue Message (Single).vi"("Priority Message? (F)"=w123, "error in (no error)"=w120, "Message"=w122, "Message Queue"=w130) -> ("error out"=w129:errorcluster)  [unwired: 1 in, 6 out]
        n84 = call "Enqueue Message (Single).vi"("Priority Message? (F)"=w123, "error in (no error)"=w120, "Message"=w122, "Message Queue"=w126) -> ("error out"=w125:errorcluster)  [unwired: 1 in, 6 out]
        n85 = call "Enqueue Message (Single).vi"("Priority Message? (F)"=w123, "error in (no error)"=w120, "Message"=w122, "Message Queue"=w119) -> ("error out"=w121:errorcluster)  [unwired: 1 in, 6 out]
        n86 = Merge Errors(w127, w128, w129, w125, w121) -> (w118:errorcluster)
        n87 = Merge Errors(w118, w137) -> (w152:errorcluster)
      }
      frame "----- Other UI Events -----" {
        # "Other UI Events"
      }
      frame "Other UI - Update Status" {
        n88 = Variant To Data(error in=w160, type="", Variant=w159) -> (data=→"Last Operation":string, error out=w157:errorcluster)
      }
      frame "----- Labram HR Events -----" {
        # "Labram HR Events"
      }
      frame "LabramHR - Set Laser" {
        # "Handle the change of Excitation Wavelength"
        n89 = Variant To Data(error in=w168, type=Laser."633 nm" ("NewVal"), Variant=w172) -> (data=w163:T29, error out=w167:errorcluster)
        n90 = Bundle By Name(cluster=T27 {"Laser Settings"={"Laser Wavelength"=enum."633 nm", "Neutral Density Filter"=enum."1%"}, "Spectrometer Settings"={"Confocal Hole Size (µm)"=150.0, "Grating"=1, "Detector"=enum."InGaAs Array"}, "Acquisition Settings"={"Acquisition Mode"=enum."Single Window", "Spectal Position (nm)"=480.0, "From (nm)"=632.0, "To (nm)"=1000.0, "Integration Time (s)"=3.0, "Number of Accumulations"=3, "AutoScanning"=FALSE, "Spike Removal"=FALSE}, "Path"=path ""} ("LabramHR"), "Laser Settings.Laser Wavelength"=w163) -> (w165:T27)
        n91 = Unbundle By Name(w171) -> ("Optical Spectrometer"=w170:refnum<queue>)
        n92 = call "Enqueue Message (Single).vi"("error in (no error)"=w167, "Message Data"=w165, "Message"="Set Laser", "Message Queue"=w170) -> ("error out"=w166:errorcluster)  [unwired: 7 out]
      }
      frame "LabramHR - Set Filter" {
        # "Handle the change of Neutral Density Filter"
        n93 = Variant To Data(error in=w183, type=Filter."1%" ("NewVal"), Variant=w182) -> (data=w174:T30, error out=w180:errorcluster)
        n94 = Bundle By Name(cluster=T27 {"Laser Settings"={"Laser Wavelength"=enum."633 nm", "Neutral Density Filter"=enum."1%"}, "Spectrometer Settings"={"Confocal Hole Size (µm)"=150.0, "Grating"=1, "Detector"=enum."InGaAs Array"}, "Acquisition Settings"={"Acquisition Mode"=enum."Single Window", "Spectal Position (nm)"=480.0, "From (nm)"=632.0, "To (nm)"=1000.0, "Integration Time (s)"=3.0, "Number of Accumulations"=3, "AutoScanning"=FALSE, "Spike Removal"=FALSE}, "Path"=path ""} ("LabramHR"), "Laser Settings.Neutral Density Filter"=w174) -> (w176:T27)
        n95 = Unbundle By Name(w178) -> ("Optical Spectrometer"=w181:refnum<queue>)
        n96 = call "Enqueue Message (Single).vi"("error in (no error)"=w180, "Message Data"=w176, "Message"="Set Filter", "Message Queue"=w181) -> ("error out"=w179:errorcluster)  [unwired: 7 out]
      }
      frame "LabramHR - Set Hole" {
        # "Handle the change in Confocal hole size"
        n97 = Variant To Data(error in=w194, type=150.0 ("Confocal Hole Size (µm) 2"), Variant=w193) -> (data=w186:dbl, error out=w189:errorcluster)
        n98 = Bundle By Name(cluster=T27 {"Laser Settings"={"Laser Wavelength"=enum."633 nm", "Neutral Density Filter"=enum."1%"}, "Spectrometer Settings"={"Confocal Hole Size (µm)"=150.0, "Grating"=1, "Detector"=enum."InGaAs Array"}, "Acquisition Settings"={"Acquisition Mode"=enum."Single Window", "Spectal Position (nm)"=480.0, "From (nm)"=632.0, "To (nm)"=1000.0, "Integration Time (s)"=3.0, "Number of Accumulations"=3, "AutoScanning"=FALSE, "Spike Removal"=FALSE}, "Path"=path ""} ("LabramHR"), "Spectrometer Settings.Confocal Hole Size (µm)"=w186) -> (w185:T27)
        n99 = Unbundle By Name(w187) -> ("Optical Spectrometer"=w191:refnum<queue>)
        n100 = call "Enqueue Message (Single).vi"("error in (no error)"=w189, "Message Data"=w185, "Message"="Set Hole", "Message Queue"=w191) -> ("error out"=w190:errorcluster)  [unwired: 7 out]
      }
      frame "LabramHR - Set Grating" {
        w196 = T32 1 items=["1800 l/mm", "150 l/mm"] ("NewVal")
        # "Handle the change of grating"
        n101 = Variant To Data(error in=w205, type=w196, Variant=w204) -> (data=w198:T32, error out=w201:errorcluster)
        n102 = Bundle By Name(cluster=T27 {"Laser Settings"={"Laser Wavelength"=enum."633 nm", "Neutral Density Filter"=enum."1%"}, "Spectrometer Settings"={"Confocal Hole Size (µm)"=150.0, "Grating"=1, "Detector"=enum."InGaAs Array"}, "Acquisition Settings"={"Acquisition Mode"=enum."Single Window", "Spectal Position (nm)"=480.0, "From (nm)"=632.0, "To (nm)"=1000.0, "Integration Time (s)"=3.0, "Number of Accumulations"=3, "AutoScanning"=FALSE, "Spike Removal"=FALSE}, "Path"=path ""} ("LabramHR"), "Spectrometer Settings.Grating"=w198) -> (w197:T27)
        n103 = Unbundle By Name(w200) -> ("Optical Spectrometer"=w203:refnum<queue>)
        n104 = call "Enqueue Message (Single).vi"("error in (no error)"=w201, "Message Data"=w197, "Message"="Set Grating", "Message Queue"=w203) -> ("error out"=w202:errorcluster)  [unwired: 7 out]
      }
      frame "LabramHR - Set Detector" {
        # "Handle the change of grating"
        n105 = Variant To Data(error in=w216, type=Detector."Silicon CCD" ("NewVal"), Variant=w215) -> (data=w209:T33, error out=w212:errorcluster)
        n106 = Bundle By Name(cluster=T27 {"Laser Settings"={"Laser Wavelength"=enum."633 nm", "Neutral Density Filter"=enum."1%"}, "Spectrometer Settings"={"Confocal Hole Size (µm)"=150.0, "Grating"=1, "Detector"=enum."InGaAs Array"}, "Acquisition Settings"={"Acquisition Mode"=enum."Single Window", "Spectal Position (nm)"=480.0, "From (nm)"=632.0, "To (nm)"=1000.0, "Integration Time (s)"=3.0, "Number of Accumulations"=3, "AutoScanning"=FALSE, "Spike Removal"=FALSE}, "Path"=path ""} ("LabramHR"), "Spectrometer Settings.Detector"=w209) -> (w208:T27)
        n107 = Unbundle By Name(w211) -> ("Optical Spectrometer"=w214:refnum<queue>)
        n108 = call "Enqueue Message (Single).vi"("error in (no error)"=w212, "Message Data"=w208, "Message"="Set Detector", "Message Queue"=w214) -> ("error out"=w213:errorcluster)  [unwired: 7 out]
      }
      frame "LabramHR - Set Spectal Position" {
        # "Handle the change of Spetrometer position"
        n109 = Variant To Data(error in=w227, type=480.0 ("Spectal Position (nm) 2"), Variant=w226) -> (data=w219:dbl, error out=w221:errorcluster)
        n110 = Bundle By Name(cluster=T27 {"Laser Settings"={"Laser Wavelength"=enum."633 nm", "Neutral Density Filter"=enum."1%"}, "Spectrometer Settings"={"Confocal Hole Size (µm)"=150.0, "Grating"=1, "Detector"=enum."InGaAs Array"}, "Acquisition Settings"={"Acquisition Mode"=enum."Single Window", "Spectal Position (nm)"=480.0, "From (nm)"=632.0, "To (nm)"=1000.0, "Integration Time (s)"=3.0, "Number of Accumulations"=3, "AutoScanning"=FALSE, "Spike Removal"=FALSE}, "Path"=path ""} ("LabramHR"), "Acquisition Settings.Spectal Position (nm)"=w219) -> (w218:T27)
        n111 = Unbundle By Name(w220) -> ("Optical Spectrometer"=w224:refnum<queue>)
        n112 = call "Enqueue Message (Single).vi"("error in (no error)"=w221, "Message Data"=w218, "Message"="Set Spectal Position", "Message Queue"=w224) -> ("error out"=w223:errorcluster)  [unwired: 7 out]
      }
      frame "LabramHR - Set Acquisition Settings" {
        # "Handle the change of integration time"
        n113 = Variant To Data(error in=w238, type=T34 {"Acquisition Mode"=enum."Single Window", "Spectal Position (nm)"=480.0, "From (nm)"=632.0, "To (nm)"=1000.0, "Integration Time (s)"=3.0, "Number of Accumulations"=3, "AutoScanning"=FALSE, "Spike Removal"=FALSE} ("Acquisition Settings 2"), Variant=w237) -> (data=w231:T34, error out=w235:errorcluster)
        n114 = Bundle By Name(cluster=T27 {"Laser Settings"={"Laser Wavelength"=enum."633 nm", "Neutral Density Filter"=enum."1%"}, "Spectrometer Settings"={"Confocal Hole Size (µm)"=150.0, "Grating"=1, "Detector"=enum."InGaAs Array"}, "Acquisition Settings"={"Acquisition Mode"=enum."Single Window", "Spectal Position (nm)"=480.0, "From (nm)"=632.0, "To (nm)"=1000.0, "Integration Time (s)"=3.0, "Number of Accumulations"=3, "AutoScanning"=FALSE, "Spike Removal"=FALSE}, "Path"=path ""} ("LabramHR"), "Acquisition Settings"=w231) -> (w230:T27)
        n115 = Unbundle By Name(w232) -> ("Optical Spectrometer"=w233:refnum<queue>)
        n116 = call "Enqueue Message (Single).vi"("error in (no error)"=w235, "Message Data"=w230, "Message"="Set Acquisition Settings", "Message Queue"=w233) -> ("error out"=w236:errorcluster)  [unwired: 7 out]
      }
      frame "LabramHR - Acquire Spectrum" {
        n117 = Unbundle By Name(w240) -> ("Optical Spectrometer"=w241:refnum<queue>)
        n118 = call "Enqueue Message (Single).vi"("error in (no error)"=w242, "Message"="Acquire Spectrum", "Message Queue"=w241) -> ("error out"=w239:errorcluster)  [unwired: 1 in, 7 out]
      }
      frame "LabramHR - Save Spectrum" {
        n119 = Unbundle By Name(w245) -> ("Optical Spectrometer"=w246:refnum<queue>)
        n120 = call "Enqueue Message (Single).vi"("error in (no error)"=w247, "Message"="Save Optical Spectrum", "Message Queue"=w246) -> ("error out"=w244:errorcluster)  [unwired: 1 in, 7 out]
      }
      frame "----- Switches & Mirrors Events -----" {
        # "Switches & Mirrors EVENTS"
      }
      frame "Switches & Mirrors - Update Visa Session" {
        n121 = Variant To Data(error in=w257, type=refnum<visa-resource-name> "COM1" ("Laser Video VISA Session 2"), Variant=w253) -> (data=w252:refnum<visa-resource-name>, error out=w255:errorcluster)
        n122 = Bundle By Name(cluster=T35 {"Relay VISA Session"="COM1", "Switches"={"Laser"=FALSE, "Video"=FALSE}, "Delays (ms)"={"Laser"=500, "Video"=1500}} ("Laser-Video Config"), "Relay VISA Session"=w252) -> (w251:T35)
        n123 = Unbundle By Name(w258) -> ("Switches & Mirrors"=w259:refnum<queue>)
        n124 = call "Enqueue Message (Single).vi"("error in (no error)"=w255, "Message Data"=w251, "Message"="Update VISA Session", "Message Queue"=w259) -> ("error out"=w260:errorcluster)  [unwired: 7 out]
      }
      frame "Switches & Mirrors - Update Laser" {
        n125 = Variant To Data(error in=w270, type=FALSE ("Laser"), Variant=w271) -> (data=w261:bool, error out=w268:errorcluster)
        n126 = Bundle By Name(cluster=T35 {"Relay VISA Session"="COM1", "Switches"={"Laser"=FALSE, "Video"=FALSE}, "Delays (ms)"={"Laser"=500, "Video"=1500}} ("Laser-Video Config"), "Switches.Laser"=w261) -> (w264:T35)
        n127 = Unbundle By Name(w266) -> ("Switches & Mirrors"=w267:refnum<queue>)
        n128 = call "Enqueue Message (Single).vi"("error in (no error)"=w268, "Message Data"=w264, "Message"="Update Laser", "Message Queue"=w267) -> ("error out"=w269:errorcluster)  [unwired: 7 out]
      }
      frame "Switches & Mirrors - Update Video" {
        n129 = Variant To Data(error in=w281, type=FALSE ("Laser"), Variant=w282) -> (data=w272:bool, error out=w279:errorcluster)
        n130 = Bundle By Name(cluster=T35 {"Relay VISA Session"="COM1", "Switches"={"Laser"=FALSE, "Video"=FALSE}, "Delays (ms)"={"Laser"=500, "Video"=1500}} ("Laser-Video Config"), "Switches.Video"=w272) -> (w275:T35)
        n131 = Unbundle By Name(w277) -> ("Switches & Mirrors"=w278:refnum<queue>)
        n132 = call "Enqueue Message (Single).vi"("error in (no error)"=w279, "Message Data"=w275, "Message"="Update Video", "Message Queue"=w278) -> ("error out"=w280:errorcluster)  [unwired: 7 out]
      }
      frame "----- Camera Events -----" {
        # "uEye Camera EVENTS"
      }
      frame "Camera - Update Settings" {
        w286 = T37 {"Settings"={"Pixel clock"=20, "Frame rate"=30.0, "Exposure time"=33.21525, "Master Gain"=0, "Red Gain"=0, "Green Gain"=0, "Blue Gain"=0, "Auto Gain"=FALSE, "White-balance"=FALSE, "Color Correction"=FALSE}} ("Camera Configuration")
        n133 = Unbundle By Name(w286) -> ("Settings"=w287:T38)
        n134 = Variant To Data(error in=w293, type=w287, Variant=w294) -> (data=w284:T38, error out=w288:errorcluster)
        n135 = Bundle By Name(cluster=w286, "Settings"=w284) -> (w285:T37)
        n136 = Unbundle By Name(w290) -> ("Camera"=w291:refnum<queue>)
        n137 = call "Enqueue Message (Single).vi"("error in (no error)"=w288, "Message Data"=w285, "Message"="Update Settings", "Message Queue"=w291) -> ("error out"=w292:errorcluster)  [unwired: 7 out]
      }
      frame "Camera - Start Live" {
        n138 = Unbundle By Name(w297) -> ("Camera"=w298:refnum<queue>)
        n139 = call "Enqueue Message (Single).vi"("error in (no error)"=w295, "Message"="Start Live", "Message Queue"=w298) -> ("error out"=w299:errorcluster)  [unwired: 1 in, 7 out]
      }
      frame "Camera - Stop Live" {
        n140 = Unbundle By Name(w302) -> ("Camera"=w303:refnum<queue>)
        n141 = call "Enqueue Message (Single).vi"("error in (no error)"=w300, "Message"="Stop Live", "Message Queue"=w303) -> ("error out"=w304:errorcluster)  [unwired: 1 in, 7 out]
      }
      frame "----- Stress Control Events -----" {
        # "Stress Control Events"
      }
      frame "Stress Control - Set UI" {
        n142 = Variant To Data(error in=w311, type=T26 {"Stress Control VISA Session"="", "Axis"=1, "Motion"=0, "Destination (°)"=0.0, "Speed (°/s)"=4.0, "Position (°)"=0.0} ("Stress Control Configuration"), Variant=w309) -> (data=w308:T26, error out=w310:errorcluster)
        n143 = Unbundle By Name(w308) -> ("Motion"=w313:u16, "Destination (°)"=w312:dbl, "Position (°)"=→"Position (°)":dbl)
        n144 = property on="Mechanism Motion" class="Ring (strict)"("Value"=w313) -> ()  [unwired: 2 in, 2 out]
        n145 = property on="Destination (°)" class="DigNum (strict)"("Value"=w312) -> ()  [unwired: 2 in, 2 out]
      }
      frame "Stress Control - Update Refnums" {
        n146 = control-ref of="Position (°)"() -> (w325:refnum<vi>)
        n147 = control-ref of="Mechanism Motion"() -> (w324:refnum<vi>)
        n148 = control-ref of="Destination (°)"() -> (w323:refnum<vi>)
        n149 = control-ref of="Stop"() -> (w317:refnum<vi>)
        n150 = control-ref of="Instrument Status"() -> (w314:refnum<vi>)
        n151 = Bundle By Name(cluster=T59 {"Instrument Status"=refnum, "Position"=refnum, "Mecahnism Motion"=refnum, "Destination"=refnum, "Apply Stress"=refnum, "Stop"=refnum, "Stress Control VISA"=refnum} ("Stress Control Refnums"), "Instrument Status"=w314, "Position"=w325, "Mecahnism Motion"=w324, "Destination"=w323, "Stop"=w317) -> (w316:T59)
        n152 = Unbundle By Name(w318) -> ("Stress Control"=w319:refnum<queue>)
        n153 = call "Enqueue Message (Single).vi"("error in (no error)"=w322, "Message Data"=w316, "Message"="Update Refnums", "Message Queue"=w319) -> ("error out"=w321:errorcluster)  [unwired: 7 out]
      }
      frame "Stress Control - Update VISA Session" {
        n154 = Variant To Data(error in=w336, type=refnum<visa-resource-name> "StrainMotor" ("Stress Controller VISA Session 2"), Variant=w329) -> (data=w328:refnum<visa-resource-name>, error out=w331:errorcluster)
        n155 = Bundle By Name(cluster=T26 {"Stress Control VISA Session"="", "Axis"=1, "Motion"=0, "Destination (°)"=0.0, "Speed (°/s)"=4.0, "Position (°)"=0.0} ("Stress Control Configuration"), "Stress Control VISA Session"=w328) -> (w327:T26)
        n156 = Unbundle By Name(w332) -> ("Stress Control"=w333:refnum<queue>)
        n157 = call "Enqueue Message (Single).vi"("error in (no error)"=w331, "Message Data"=w327, "Message"="Update Visa Session", "Message Queue"=w333) -> ("error out"=w335:errorcluster)  [unwired: 7 out]
      }
      frame "Stress Control - Update Configuration" {
        n158 = Variant To Data(error in=w347, type=4.0 ("Speed (°/s) 2"), Variant=w341) -> (data=w339:dbl, error out=w342:errorcluster)
        n159 = Bundle By Name(cluster=T26 {"Stress Control VISA Session"="", "Axis"=1, "Motion"=0, "Destination (°)"=0.0, "Speed (°/s)"=4.0, "Position (°)"=0.0} ("Stress Control Configuration"), "Speed (°/s)"=w339) -> (w338:T26)
        n160 = Unbundle By Name(w343) -> ("Stress Control"=w344:refnum<queue>)
        n161 = call "Enqueue Message (Single).vi"("error in (no error)"=w342, "Message Data"=w338, "Message"="Update Configuration", "Message Queue"=w344) -> ("error out"=w346:errorcluster)  [unwired: 7 out]
      }
      frame "Stress Control - Update Motion Mode" {
        w351 = u16 0 items=["Absolute", "Relative"] ("Motion 2")
        n162 = Variant To Data(error in=w358, type=w351, Variant=w352) -> (data=w350:u16, error out=w353:errorcluster)
        n163 = Bundle By Name(cluster=T26 {"Stress Control VISA Session"="", "Axis"=1, "Motion"=0, "Destination (°)"=0.0, "Speed (°/s)"=4.0, "Position (°)"=0.0} ("Stress Control Configuration"), "Motion"=w350) -> (w349:T26)
        n164 = Unbundle By Name(w354) -> ("Stress Control"=w355:refnum<queue>)
        n165 = call "Enqueue Message (Single).vi"("error in (no error)"=w353, "Message Data"=w349, "Message"="Update Motion Mode", "Message Queue"=w355) -> ("error out"=w357:errorcluster)  [unwired: 7 out]
      }
      frame "Stress Control - Update Destination" {
        n166 = Variant To Data(error in=w369, type=0.0 ("Destination (°) 2"), Variant=w363) -> (data=w362:dbl, error out=w364:errorcluster)
        n167 = Bundle By Name(cluster=T26 {"Stress Control VISA Session"="", "Axis"=1, "Motion"=0, "Destination (°)"=0.0, "Speed (°/s)"=4.0, "Position (°)"=0.0} ("Stress Control Configuration"), "Destination (°)"=w362) -> (w360:T26)
        n168 = Unbundle By Name(w365) -> ("Stress Control"=w366:refnum<queue>)
        n169 = call "Enqueue Message (Single).vi"("error in (no error)"=w364, "Message Data"=w360, "Message"="Update Destination", "Message Queue"=w366) -> ("error out"=w368:errorcluster)  [unwired: 7 out]
      }
      frame "Stress Control - Change Stress" {
        n170 = Unbundle By Name(w372) -> ("Stress Control"=w373:refnum<queue>)
        n171 = call "Enqueue Message (Single).vi"("error in (no error)"=w370, "Message"="Change Stress", "Message Queue"=w373) -> ("error out"=w374:errorcluster)  [unwired: 1 in, 7 out]
      }
      frame "----- Parameter Analyzer Events -----" {
        # "Parameter Analyzer Events"
      }
      frame "Parameter Analyzer - Update Visa Session" {
        w377 = T17 {"Parameter Analyzer VISA Session"="COM1", "Sweeping Time Parameters"={"Integration Time"=0, "Short Integration Time (s)"=0.0, "Long Integration Time (s)"=0.0, "Wait Time Parameter"=1.0}, "Acquisition Mode"=enum."Sweeping Mode", "Status Polling Time (ms)"=1000, "Comment"="Test VI", "SMU 1 - Sweeping"={"Start / Offset"=0.0, "Stop / Ratio"=1.0, "Step \n(linear only)"=0.01, "Compliance"=0.1, "Power \nCompliance"=0.0, "Mode"=0, "Function"=0, "Sweep Mode"=FALSE}, "SMU 2 - Sweeping"={"Start / Offset"=0.0, "Stop / Ratio"=1.0, "Step \n(linear only)"=0.01, "Compliance"=0.1, "Power \nCompliance"=0.0, "Mode"=0, "Function"=0, "Sweep Mode"=FALSE}, "SMU 3 - Sweeping"={"Start / Offset"=0.0, "Stop / Ratio"=1.0, "Step \n(linear only)"=0.01, "Compliance"=0.1, "Power \nCompliance"=0.0, "Mode"=0, "Function"=0, "Sweep Mode"=FALSE}, "SMU 4 - Sweeping"={"Start / Offset"=0.0, "Stop / Ratio"=1.0, "Step \n(linear only)"=0.01, "Compliance"=0.1, "Power \nCompliance"=0.0, "Mode"=1, "Function"=0, "Sweep Mode"=FALSE}, "Sweep Spacing"=0, "Range"=0, "SMU1 - Sampling"={"Source"=10.0, "Compliance"=1e-05, "Mode"=0, "Function"=FALSE}, "SMU2 - Sampling"={"Source"=10.0, "Compliance"=1e-05, "Mode"=0, "Function"=FALSE}, "SMU3 - Sampling"={"Source"=10.0, "Compliance"=1e-05, "Mode"=0, "Function"=FALSE}, "SMU4 - Sampling"={"Source"=10.0, "Compliance"=1e-05, "Mode"=0, "Function"=FALSE}, "Sampling Time Parameters"={"Initial Interval (s)"=0.1, "Number of Samples"=60, "Total Sampling Time (s)"=10.0, "Hold Time (s)"=0.0, "Sampling Mode"=0, "Sampling Time"=0}, "Stop Condition"={"Enable Delay (s)"=0.0, "Name"="", "Threshold"=0.0, "num. of events"=1, "Event"=0, "Stop Condition Enable"=FALSE}} ("HP4155C Configuration")
        n172 = Unbundle By Name(w377) -> ("Parameter Analyzer VISA Session"=w378:refnum<visa-resource-name>)
        n173 = Variant To Data(error in=w386, type=w378, Variant=w385) -> (data=w376:refnum<visa-resource-name>, error out=w381:errorcluster)
        n174 = Bundle By Name(cluster=w377, "Parameter Analyzer VISA Session"=w376) -> (w379:T17)
        n175 = Unbundle By Name(w382) -> ("Parameter Analyzer"=w383:refnum<queue>)
        n176 = call "Enqueue Message (Single).vi"("error in (no error)"=w381, "Message Data"=w379, "Message"="Update Visa Session", "Message Queue"=w383) -> ("error out"=w380:errorcluster)  [unwired: 7 out]
      }
      frame "Parameter Analyzer - Configure Integration time" {
        w387 = T17 {"Parameter Analyzer VISA Session"="COM1", "Sweeping Time Parameters"={"Integration Time"=0, "Short Integration Time (s)"=0.0, "Long Integration Time (s)"=0.0, "Wait Time Parameter"=1.0}, "Acquisition Mode"=enum."Sweeping Mode", "Status Polling Time (ms)"=1000, "Comment"="Test VI", "SMU 1 - Sweeping"={"Start / Offset"=0.0, "Stop / Ratio"=1.0, "Step \n(linear only)"=0.01, "Compliance"=0.1, "Power \nCompliance"=0.0, "Mode"=0, "Function"=0, "Sweep Mode"=FALSE}, "SMU 2 - Sweeping"={"Start / Offset"=0.0, "Stop / Ratio"=1.0, "Step \n(linear only)"=0.01, "Compliance"=0.1, "Power \nCompliance"=0.0, "Mode"=0, "Function"=0, "Sweep Mode"=FALSE}, "SMU 3 - Sweeping"={"Start / Offset"=0.0, "Stop / Ratio"=1.0, "Step \n(linear only)"=0.01, "Compliance"=0.1, "Power \nCompliance"=0.0, "Mode"=0, "Function"=0, "Sweep Mode"=FALSE}, "SMU 4 - Sweeping"={"Start / Offset"=0.0, "Stop / Ratio"=1.0, "Step \n(linear only)"=0.01, "Compliance"=0.1, "Power \nCompliance"=0.0, "Mode"=1, "Function"=0, "Sweep Mode"=FALSE}, "Sweep Spacing"=0, "Range"=0, "SMU1 - Sampling"={"Source"=10.0, "Compliance"=1e-05, "Mode"=0, "Function"=FALSE}, "SMU2 - Sampling"={"Source"=10.0, "Compliance"=1e-05, "Mode"=0, "Function"=FALSE}, "SMU3 - Sampling"={"Source"=10.0, "Compliance"=1e-05, "Mode"=0, "Function"=FALSE}, "SMU4 - Sampling"={"Source"=10.0, "Compliance"=1e-05, "Mode"=0, "Function"=FALSE}, "Sampling Time Parameters"={"Initial Interval (s)"=0.1, "Number of Samples"=60, "Total Sampling Time (s)"=10.0, "Hold Time (s)"=0.0, "Sampling Mode"=0, "Sampling Time"=0}, "Stop Condition"={"Enable Delay (s)"=0.0, "Name"="", "Threshold"=0.0, "num. of events"=1, "Event"=0, "Stop Condition Enable"=FALSE}} ("HP4155C Configuration")
        n177 = Unbundle By Name(w387) -> ("Sweeping Time Parameters"=w388:T18)
        n178 = Variant To Data(error in=w397, type=w388, Variant=w396) -> (data=w389:T18, error out=w393:errorcluster)
        n179 = Bundle By Name(cluster=w387, "Sweeping Time Parameters"=w389) -> (w390:T17)
        n180 = Unbundle By Name(w391) -> ("Parameter Analyzer"=w394:refnum<queue>)
        n181 = call "Enqueue Message (Single).vi"("error in (no error)"=w393, "Message Data"=w390, "Message"="Configure Integration Time", "Message Queue"=w394) -> ("error out"=w392:errorcluster)  [unwired: 7 out]
      }
      frame "Parameter Analyzer - Configure Sweeping" {
        n182 = Variant To Data(error in=w414, type=T60 {"SMU 1 - Sweeping"={"Start / Offset"=0.0, "Stop / Ratio"=0.0, "Step (linear only)"=0.0, "Compliance"=0.0, "Power Compliance"=0.0, "Mode"=0, "Function"=0, "Sweep Mode"=FALSE}, "SMU 2 - Sweeping"={"Start / Offset"=0.0, "Stop / Ratio"=0.0, "Step (linear only)"=0.0, "Compliance"=0.0, "Power Compliance"=0.0, "Mode"=0, "Function"=0, "Sweep Mode"=FALSE}, "SMU 3 - Sweeping"={"Start / Offset"=0.0, "Stop / Ratio"=0.0, "Step (linear only)"=0.0, "Compliance"=0.0, "Power Compliance"=0.0, "Mode"=0, "Function"=0, "Sweep Mode"=FALSE}, "SMU 4 - Sweeping"={"Start / Offset"=0.0, "Stop / Ratio"=0.0, "Step (linear only)"=0.0, "Compliance"=0.0, "Power Compliance"=0.0, "Mode"=0, "Function"=0, "Sweep Mode"=FALSE}, "Sweep Spacing"=0, "Range"=0} ("output cluster"), Variant=w413) -> (data=w412:T60, error out=w404:errorcluster)
        n183 = Unbundle By Name(w412) -> ("SMU 1 - Sweeping"=w407:T63, "SMU 2 - Sweeping"=w408:T63, "SMU 3 - Sweeping"=w409:T63, "SMU 4 - Sweeping"=w410:T63, "Sweep Spacing"=w411:u16, "Range"=w401:u16)
        n184 = Bundle By Name(cluster=T17 {"Parameter Analyzer VISA Session"="COM1", "Sweeping Time Parameters"={"Integration Time"=0, "Short Integration Time (s)"=0.0, "Long Integration Time (s)"=0.0, "Wait Time Parameter"=1.0}, "Acquisition Mode"=enum."Sweeping Mode", "Status Polling Time (ms)"=1000, "Comment"="Test VI", "SMU 1 - Sweeping"={"Start / Offset"=0.0, "Stop / Ratio"=1.0, "Step \n(linear only)"=0.01, "Compliance"=0.1, "Power \nCompliance"=0.0, "Mode"=0, "Function"=0, "Sweep Mode"=FALSE}, "SMU 2 - Sweeping"={"Start / Offset"=0.0, "Stop / Ratio"=1.0, "Step \n(linear only)"=0.01, "Compliance"=0.1, "Power \nCompliance"=0.0, "Mode"=0, "Function"=0, "Sweep Mode"=FALSE}, "SMU 3 - Sweeping"={"Start / Offset"=0.0, "Stop / Ratio"=1.0, "Step \n(linear only)"=0.01, "Compliance"=0.1, "Power \nCompliance"=0.0, "Mode"=0, "Function"=0, "Sweep Mode"=FALSE}, "SMU 4 - Sweeping"={"Start / Offset"=0.0, "Stop / Ratio"=1.0, "Step \n(linear only)"=0.01, "Compliance"=0.1, "Power \nCompliance"=0.0, "Mode"=1, "Function"=0, "Sweep Mode"=FALSE}, "Sweep Spacing"=0, "Range"=0, "SMU1 - Sampling"={"Source"=10.0, "Compliance"=1e-05, "Mode"=0, "Function"=FALSE}, "SMU2 - Sampling"={"Source"=10.0, "Compliance"=1e-05, "Mode"=0, "Function"=FALSE}, "SMU3 - Sampling"={"Source"=10.0, "Compliance"=1e-05, "Mode"=0, "Function"=FALSE}, "SMU4 - Sampling"={"Source"=10.0, "Compliance"=1e-05, "Mode"=0, "Function"=FALSE}, "Sampling Time Parameters"={"Initial Interval (s)"=0.1, "Number of Samples"=60, "Total Sampling Time (s)"=10.0, "Hold Time (s)"=0.0, "Sampling Mode"=0, "Sampling Time"=0}, "Stop Condition"={"Enable Delay (s)"=0.0, "Name"="", "Threshold"=0.0, "num. of events"=1, "Event"=0, "Stop Condition Enable"=FALSE}} ("HP4155C Configuration"), "SMU 1 - Sweeping"=w407, "SMU 2 - Sweeping"=w408, "SMU 3 - Sweeping"=w409, "SMU 4 - Sweeping"=w410, "Sweep Spacing"=w411, "Range"=w401) -> (w400:T17)
        n185 = Unbundle By Name(w402) -> ("Parameter Analyzer"=w405:refnum<queue>)
        n186 = call "Enqueue Message (Single).vi"("error in (no error)"=w404, "Message Data"=w400, "Message"="Configure Sweeping", "Message Queue"=w405) -> ("error out"=w403:errorcluster)  [unwired: 7 out]
      }
      frame "Parameter Analyzer - Configure Sampling" {
        n187 = Variant To Data(error in=w431, type=T61 {"SMU1 - Sampling"={"Source"=0.0, "Compliance"=0.0, "Mode"=0, "Function"=FALSE}, "SMU2 - Sampling"={"Source"=0.0, "Compliance"=0.0, "Mode"=0, "Function"=FALSE}, "SMU3 - Sampling"={"Source"=0.0, "Compliance"=0.0, "Mode"=0, "Function"=FALSE}, "SMU4 - Sampling"={"Source"=0.0, "Compliance"=0.0, "Mode"=0, "Function"=FALSE}, "Sampling Parameters"={"Initial Interval (s)"=0.0, "Number of Samples"=0, "Total Sampling Time (s)"=0.0, "Hold Time (s)"=0.0, "Sampling Mode"=0, "Sampling Time"=0}, "Stop Condition"={"Enable Delay (s)"=0.0, "Name"="", "Threshold"=0.0, "num. of events"=0, "Event"=0, "Stop Condition Enable"=FALSE}} ("output cluster"), Variant=w430) -> (data=w429:T61, error out=w424:errorcluster)
        n188 = Unbundle By Name(w429) -> ("SMU1 - Sampling"=w420:T64, "SMU2 - Sampling"=w419:T64, "SMU3 - Sampling"=w418:T64, "SMU4 - Sampling"=w417:T64, "Sampling Parameters"=w428:T65, "Stop Condition"=w427:T66)
        n189 = Bundle By Name(cluster=T17 {"Parameter Analyzer VISA Session"="COM1", "Sweeping Time Parameters"={"Integration Time"=0, "Short Integration Time (s)"=0.0, "Long Integration Time (s)"=0.0, "Wait Time Parameter"=1.0}, "Acquisition Mode"=enum."Sweeping Mode", "Status Polling Time (ms)"=1000, "Comment"="Test VI", "SMU 1 - Sweeping"={"Start / Offset"=0.0, "Stop / Ratio"=1.0, "Step \n(linear only)"=0.01, "Compliance"=0.1, "Power \nCompliance"=0.0, "Mode"=0, "Function"=0, "Sweep Mode"=FALSE}, "SMU 2 - Sweeping"={"Start / Offset"=0.0, "Stop / Ratio"=1.0, "Step \n(linear only)"=0.01, "Compliance"=0.1, "Power \nCompliance"=0.0, "Mode"=0, "Function"=0, "Sweep Mode"=FALSE}, "SMU 3 - Sweeping"={"Start / Offset"=0.0, "Stop / Ratio"=1.0, "Step \n(linear only)"=0.01, "Compliance"=0.1, "Power \nCompliance"=0.0, "Mode"=0, "Function"=0, "Sweep Mode"=FALSE}, "SMU 4 - Sweeping"={"Start / Offset"=0.0, "Stop / Ratio"=1.0, "Step \n(linear only)"=0.01, "Compliance"=0.1, "Power \nCompliance"=0.0, "Mode"=1, "Function"=0, "Sweep Mode"=FALSE}, "Sweep Spacing"=0, "Range"=0, "SMU1 - Sampling"={"Source"=10.0, "Compliance"=1e-05, "Mode"=0, "Function"=FALSE}, "SMU2 - Sampling"={"Source"=10.0, "Compliance"=1e-05, "Mode"=0, "Function"=FALSE}, "SMU3 - Sampling"={"Source"=10.0, "Compliance"=1e-05, "Mode"=0, "Function"=FALSE}, "SMU4 - Sampling"={"Source"=10.0, "Compliance"=1e-05, "Mode"=0, "Function"=FALSE}, "Sampling Time Parameters"={"Initial Interval (s)"=0.1, "Number of Samples"=60, "Total Sampling Time (s)"=10.0, "Hold Time (s)"=0.0, "Sampling Mode"=0, "Sampling Time"=0}, "Stop Condition"={"Enable Delay (s)"=0.0, "Name"="", "Threshold"=0.0, "num. of events"=1, "Event"=0, "Stop Condition Enable"=FALSE}} ("HP4155C Configuration"), "SMU1 - Sampling"=w420, "SMU2 - Sampling"=w419, "SMU3 - Sampling"=w418, "SMU4 - Sampling"=w417, "Sampling Time Parameters"=w428, "Stop Condition"=w427) -> (w421:T17)
        n190 = Unbundle By Name(w422) -> ("Parameter Analyzer"=w425:refnum<queue>)
        n191 = call "Enqueue Message (Single).vi"("error in (no error)"=w424, "Message Data"=w421, "Message"="Configure Sampling", "Message Queue"=w425) -> ("error out"=w423:errorcluster)  [unwired: 7 out]
      }
      frame "Parameter Analyzer - Save Measurement" {
        n192 = Unbundle By Name(w433) -> ("Parameter Analyzer"=w435:refnum<queue>)
        n193 = call "Enqueue Message (Single).vi"("error in (no error)"=w432, "Message"="Save Electrical Measurement", "Message Queue"=w435) -> ("error out"=w434:errorcluster)  [unwired: 1 in, 7 out]
      }
      frame "----- Switching Matrix Events ----- " {
        # "Switching Matrix Events"
      }
      frame "Switching Matrix - Update Visa Session" {
        w438 = T25 {"Switching Matrix VISA Session"="GPIB0::18::INSTR", "Connections"=[{"Connections"=[FALSE, FALSE, FALSE, FALSE, FALSE, FALSE, FALSE, FALSE, FALSE, FALSE, FALSE, FALSE], "Connection Type"=enum."Disconnected"}, {"Connections"=[FALSE, FALSE, FALSE, FALSE, FALSE, FALSE, FALSE, FALSE, FALSE, FALSE, FALSE, FALSE], "Connection Type"=enum."Disconnected"}, {"Connections"=[FALSE, FALSE, FALSE, FALSE, FALSE, FALSE, FALSE, FALSE, FALSE, FALSE, FALSE, FALSE], "Connection Type"=enum."Disconnected"}, {"Connections"=[FALSE, FALSE, FALSE, FALSE, FALSE, FALSE, FALSE, FALSE, FALSE, FALSE, FALSE, FALSE], "Connection Type"=enum."Disconnected"}, {"Connections"=[FALSE, FALSE, FALSE, FALSE, FALSE, FALSE, FALSE, FALSE, FALSE, FALSE, FALSE, FALSE], "Connection Type"=enum."Disconnected"}, {"Connections"=[FALSE, FALSE, FALSE, FALSE, FALSE, FALSE, FALSE, FALSE, FALSE, FALSE, FALSE, FALSE], "Connection Type"=enum."Disconnected"}, {"Connections"=[FALSE, FALSE, FALSE, FALSE, FALSE, FALSE, FALSE, FALSE, FALSE, FALSE, FALSE, FALSE], "Connection Type"=enum."Disconnected"}, {"Connections"=[FALSE, FALSE, FALSE, FALSE, FALSE, FALSE, FALSE, FALSE, FALSE, FALSE, FALSE, FALSE], "Connection Type"=enum."Disconnected"}]} ("Keythley 707A Switching Matrix Configuration")
        n194 = Unbundle By Name(w438) -> ("Switching Matrix VISA Session"=w439:refnum<visa-resource-name>)
        n195 = Variant To Data(error in=w445, type=w439, Variant=w442) -> (data=w441:refnum<visa-resource-name>, error out=w443:errorcluster)
        n196 = Bundle By Name(cluster=w438, "Switching Matrix VISA Session"=w441) -> (w440:T25)
        n197 = Unbundle By Name(w446) -> ("Switching Matrix"=w447:refnum<queue>)
        n198 = call "Enqueue Message (Single).vi"("error in (no error)"=w443, "Message Data"=w440, "Message"="Update Visa Session", "Message Queue"=w447) -> ("error out"=w448:errorcluster)  [unwired: 7 out]
      }
      frame "Switching Matrix - Set Connections" {
        w449 = T25 {"Switching Matrix VISA Session"="GPIB0::18::INSTR", "Connections"=[{"Connections"=[FALSE, FALSE, FALSE, FALSE, FALSE, FALSE, FALSE, FALSE, FALSE, FALSE, FALSE, FALSE], "Connection Type"=enum."Disconnected"}, {"Connections"=[FALSE, FALSE, FALSE, FALSE, FALSE, FALSE, FALSE, FALSE, FALSE, FALSE, FALSE, FALSE], "Connection Type"=enum."Disconnected"}, {"Connections"=[FALSE, FALSE, FALSE, FALSE, FALSE, FALSE, FALSE, FALSE, FALSE, FALSE, FALSE, FALSE], "Connection Type"=enum."Disconnected"}, {"Connections"=[FALSE, FALSE, FALSE, FALSE, FALSE, FALSE, FALSE, FALSE, FALSE, FALSE, FALSE, FALSE], "Connection Type"=enum."Disconnected"}, {"Connections"=[FALSE, FALSE, FALSE, FALSE, FALSE, FALSE, FALSE, FALSE, FALSE, FALSE, FALSE, FALSE], "Connection Type"=enum."Disconnected"}, {"Connections"=[FALSE, FALSE, FALSE, FALSE, FALSE, FALSE, FALSE, FALSE, FALSE, FALSE, FALSE, FALSE], "Connection Type"=enum."Disconnected"}, {"Connections"=[FALSE, FALSE, FALSE, FALSE, FALSE, FALSE, FALSE, FALSE, FALSE, FALSE, FALSE, FALSE], "Connection Type"=enum."Disconnected"}, {"Connections"=[FALSE, FALSE, FALSE, FALSE, FALSE, FALSE, FALSE, FALSE, FALSE, FALSE, FALSE, FALSE], "Connection Type"=enum."Disconnected"}]} ("Keythley 707A Switching Matrix Configuration")
        n199 = Unbundle By Name(w449) -> ("Connections"=w450:T67)
        n200 = Variant To Data(error in=w456, type=w450, Variant=w453) -> (data=w452:T67, error out=w454:errorcluster)
        n201 = Bundle By Name(cluster=w449, "Connections"=w452) -> (w451:T25)
        n202 = Unbundle By Name(w457) -> ("Switching Matrix"=w458:refnum<queue>)
        n203 = call "Enqueue Message (Single).vi"("error in (no error)"=w454, "Message Data"=w451, "Message"="Set Connections", "Message Queue"=w458) -> ("error out"=w459:errorcluster)  [unwired: 7 out]
      }
      frame "Switching Matrix - Disconnect All" {
        n204 = Unbundle By Name(w462) -> ("Switching Matrix"=w463:refnum<queue>)
        n205 = call "Enqueue Message (Single).vi"("error in (no error)"=w460, "Message"="Disconnect All", "Message Queue"=w463) -> ("error out"=w464:errorcluster)  [unwired: 1 in, 7 out]
      }
      frame "Switching Matrix - Ground All" {
        n206 = Unbundle By Name(w467) -> ("Switching Matrix"=w468:refnum<queue>)
        n207 = call "Enqueue Message (Single).vi"("error in (no error)"=w465, "Message"="Ground All", "Message Queue"=w468) -> ("error out"=w469:errorcluster)  [unwired: 1 in, 7 out]
      }
      frame "----- XYZ Stage Events -----" {
        # "NEW DEVICE EVENTS"
      }
      frame "XYZ Stage - Update Visa Session" {
        w471 = T39 {"Connection Settings"={"Tango VISA"="", "Baudrate"=57600, "Show Protocol?"=FALSE}, "Manual Control"={"North"=FALSE, "South"=FALSE, "West"=FALSE, "East"=FALSE, "Up"=FALSE, "Down"=FALSE, "Stop"=FALSE, "XY Step"=0.0, "Z step"=0.0}, "Coordinate Control"={"Motion Mode"=enum."Absolute", "Destination [mm]"=[]}} ("Configuration")
        n208 = Unbundle By Name(w471) -> ("Connection Settings.Tango VISA"=w479:refnum<visa-resource-name>)
        n209 = Variant To Data(error in=w481, type=w479, Variant=w480) -> (data=w472:refnum<visa-resource-name>, error out=w477:errorcluster)
        n210 = Bundle By Name(cluster=w471, "Connection Settings.Tango VISA"=w472) -> (w473:T39)
        n211 = Unbundle By Name(w475) -> ("XYZ Stage"=w474:refnum<queue>)
        n212 = call "Enqueue Message (Single).vi"("error in (no error)"=w477, "Message Data"=w473, "Message"="Manual Control", "Message Queue"=w474) -> ("error out"=w476:errorcluster)  [unwired: 7 out]
      }
      frame "XYZ Stage - Manual Control" {
        w483 = T39 {"Connection Settings"={"Tango VISA"="", "Baudrate"=57600, "Show Protocol?"=FALSE}, "Manual Control"={"North"=FALSE, "South"=FALSE, "West"=FALSE, "East"=FALSE, "Up"=FALSE, "Down"=FALSE, "Stop"=FALSE, "XY Step"=0.0, "Z step"=0.0}, "Coordinate Control"={"Motion Mode"=enum."Absolute", "Destination [mm]"=[]}} ("Configuration")
        n213 = Unbundle By Name(w483) -> ("Manual Control"=w482:T41)
        n214 = Variant To Data(error in=w492, type=w482, Variant=w491) -> (data=w484:T41, error out=w489:errorcluster)
        n215 = Bundle By Name(cluster=w483, "Manual Control"=w484) -> (w485:T39)
        n216 = Unbundle By Name(w487) -> ("XYZ Stage"=w486:refnum<queue>)
        n217 = call "Enqueue Message (Single).vi"("error in (no error)"=w489, "Message Data"=w485, "Message"="Manual Control", "Message Queue"=w486) -> ("error out"=w488:errorcluster)  [unwired: 7 out]
      }
      frame "----- AutoFocus Events -----" {
        # "NEW DEVICE EVENTS"
      }
      frame "AutoFocus - Set Match Criteria" {
        w494 = T43 {"Matching Criteria"={"Minimum Score"=700.0, "Color Score Weight"=57600.0, "Minimum Contrast"=50, "Match Mode"=0, "Match Feature Mode"=0, "Subpixel Accuracy"=TRUE, "Color Sensitivity"=1, "Search Strategy"=1}, "Z Scan Parameters"={"Z Range"=1380.0, "Resolution"=5000.0, "Initial Direction"=enum."Up", "Focus Threshold"=0.1, "Ascent Constant"=0.1}, "Displacement"=0.0, "Transformation Matrix"=[]} ("Configuration")
        n218 = Unbundle By Name(w494) -> ("Matching Criteria"=w502:T68)
        n219 = Variant To Data(error in=w504, type=w502, Variant=w503) -> (data=w495:T68, error out=w500:errorcluster)
        n220 = Bundle By Name(cluster=w494, "Matching Criteria"=w495) -> (w496:T43)
        n221 = Unbundle By Name(w498) -> ("AutoFocus"=w497:refnum<queue>)
        n222 = call "Enqueue Message (Single).vi"("error in (no error)"=w500, "Message Data"=w496, "Message"="Set Match Criteria", "Message Queue"=w497) -> ("error out"=w499:errorcluster)  [unwired: 7 out]
      }
      frame "AutoFocus - Link Stage & Camera" {
        w505 = T43 {"Matching Criteria"={"Minimum Score"=700.0, "Color Score Weight"=57600.0, "Minimum Contrast"=50, "Match Mode"=0, "Match Feature Mode"=0, "Subpixel Accuracy"=TRUE, "Color Sensitivity"=1, "Search Strategy"=1}, "Z Scan Parameters"={"Z Range"=1380.0, "Resolution"=5000.0, "Initial Direction"=enum."Up", "Focus Threshold"=0.1, "Ascent Constant"=0.1}, "Displacement"=0.0, "Transformation Matrix"=[]} ("Configuration")
        n223 = Unbundle By Name(w505) -> ("Displacement"=w513:dbl)
        n224 = Variant To Data(error in=w515, type=w513, Variant=w514) -> (data=w506:dbl, error out=w511:errorcluster)
        n225 = Bundle By Name(cluster=w505, "Displacement"=w506) -> (w507:T43)
        n226 = Unbundle By Name(w509) -> ("AutoFocus"=w508:refnum<queue>)
        n227 = call "Enqueue Message (Single).vi"("error in (no error)"=w511, "Message Data"=w507, "Message"="Link Stage & Camera", "Message Queue"=w508) -> ("error out"=w510:errorcluster)  [unwired: 7 out]
      }
      frame "AutoFocus - Focus" {
        w516 = T43 {"Matching Criteria"={"Minimum Score"=700.0, "Color Score Weight"=57600.0, "Minimum Contrast"=50, "Match Mode"=0, "Match Feature Mode"=0, "Subpixel Accuracy"=TRUE, "Color Sensitivity"=1, "Search Strategy"=1}, "Z Scan Parameters"={"Z Range"=1380.0, "Resolution"=5000.0, "Initial Direction"=enum."Up", "Focus Threshold"=0.1, "Ascent Constant"=0.1}, "Displacement"=0.0, "Transformation Matrix"=[]} ("Configuration")
        n228 = Unbundle By Name(w516) -> ("Z Scan Parameters"=w524:T44)
        n229 = Variant To Data(error in=w526, type=w524, Variant=w525) -> (data=w517:T44, error out=w522:errorcluster)
        n230 = Bundle By Name(cluster=w516, "Z Scan Parameters"=w517) -> (w518:T43)
        n231 = Unbundle By Name(w520) -> ("AutoFocus"=w519:refnum<queue>)
        n232 = call "Enqueue Message (Single).vi"("error in (no error)"=w522, "Message Data"=w518, "Message"="Focus", "Message Queue"=w519) -> ("error out"=w521:errorcluster)  [unwired: 7 out]
      }
      frame "AutoFocus - Set Target" {
        n233 = Unbundle By Name(w529) -> ("AutoFocus"=w528:refnum<queue>)
        n234 = call "Enqueue Message (Single).vi"("error in (no error)"=w527, "Message"="Set Target", "Message Queue"=w528) -> ("error out"=w530:errorcluster)  [unwired: 1 in, 7 out]
      }
      frame "AutoFocus - Find Target" {
        n235 = Unbundle By Name(w534) -> ("AutoFocus"=w533:refnum<queue>)
        n236 = call "Enqueue Message (Single).vi"("error in (no error)"=w532, "Message"="Find Target", "Message Queue"=w533) -> ("error out"=w535:errorcluster)  [unwired: 1 in, 7 out]
      }
      frame "AutoFocus - Align" {
        n237 = Unbundle By Name(w539) -> ("AutoFocus"=w538:refnum<queue>)
        n238 = call "Enqueue Message (Single).vi"("error in (no error)"=w537, "Message"="Align", "Message Queue"=w538) -> ("error out"=w540:errorcluster)  [unwired: 1 in, 7 out]
      }
      frame "AutoFocus - Grab Image" {
        n239 = Unbundle By Name(w544) -> ("AutoFocus"=w543:refnum<queue>)
        n240 = call "Enqueue Message (Single).vi"("error in (no error)"=w542, "Message"="Grab Image", "Message Queue"=w543) -> ("error out"=w545:errorcluster)  [unwired: 1 in, 7 out]
      }
      frame "AutoFocus - Set ROI" {
        n241 = Unbundle By Name(w549) -> ("AutoFocus"=w548:refnum<queue>)
        n242 = call "Enqueue Message (Single).vi"("error in (no error)"=w547, "Message"="Set ROI", "Message Queue"=w548) -> ("error out"=w550:errorcluster)  [unwired: 1 in, 7 out]
      }
      frame "AutoFocus - Get ROI" {
        n243 = Unbundle By Name(w554) -> ("AutoFocus"=w553:refnum<queue>)
        n244 = call "Enqueue Message (Single).vi"("error in (no error)"=w552, "Message"="Get ROI", "Message Queue"=w553) -> ("error out"=w555:errorcluster)  [unwired: 1 in, 7 out]
      }
      frame "AutoFocus - Start Tracking" {
        n245 = Unbundle By Name(w559) -> ("AutoFocus"=w558:refnum<queue>)
        n246 = call "Enqueue Message (Single).vi"("error in (no error)"=w557, "Message"="Start Tracking", "Message Queue"=w558) -> ("error out"=w560:errorcluster)  [unwired: 1 in, 7 out]
      }
      frame "AutoFocus - Stop Tracking" {
        n247 = Unbundle By Name(w564) -> ("AutoFocus"=w563:refnum<queue>)
        n248 = call "Enqueue Message (Single).vi"("error in (no error)"=w562, "Message"="Stop Tracking", "Message Queue"=w563) -> ("error out"=w565:errorcluster)  [unwired: 1 in, 7 out]
      }
      frame "----- Instrument Sequence Events -----" {
        # "NEW DEVICE EVENTS"
      }
      frame "Instrument Sequence - Add Step" {
        n249 = Unbundle By Name(w572) -> ("Instrument Sequence"=w571:refnum<queue>)
        n250 = call "Enqueue Message (Single).vi"("error in (no error)"=w570, "Message"="Add Step", "Message Queue"=w571) -> ("error out"=w569:errorcluster)  [unwired: 1 in, 7 out]
      }
      frame "Instrument Sequence - Remove Step" {
        n251 = Unbundle By Name(w577) -> ("Instrument Sequence"=w576:refnum<queue>)
        n252 = call "Enqueue Message (Single).vi"("error in (no error)"=w575, "Message"="Remove Step", "Message Queue"=w576) -> ("error out"=w574:errorcluster)  [unwired: 1 in, 7 out]
      }
      frame "Instrument Sequence - Clear Sequence" {
        n253 = Unbundle By Name(w582) -> ("Instrument Sequence"=w581:refnum<queue>)
        n254 = call "Enqueue Message (Single).vi"("error in (no error)"=w580, "Message"="Clear Sequence", "Message Queue"=w581) -> ("error out"=w579:errorcluster)  [unwired: 1 in, 7 out]
      }
      frame "Instrument Sequence - Save Sequence" {
        n255 = Unbundle By Name(w587) -> ("Instrument Sequence"=w586:refnum<queue>)
        n256 = call "Enqueue Message (Single).vi"("error in (no error)"=w585, "Message"="Save Sequence", "Message Queue"=w586) -> ("error out"=w584:errorcluster)  [unwired: 1 in, 7 out]
      }
      frame "Instrument Sequence - Load Sequence" {
        n257 = Unbundle By Name(w592) -> ("Instrument Sequence"=w591:refnum<queue>)
        n258 = call "Enqueue Message (Single).vi"("error in (no error)"=w590, "Message"="Load Sequence", "Message Queue"=w591) -> ("error out"=w589:errorcluster)  [unwired: 1 in, 7 out]
      }
      frame "Instrument Sequence - Start Sequence" {
        n259 = Unbundle By Name(w597) -> ("Instrument Sequence"=w596:refnum<queue>)
        n260 = call "Enqueue Message (Single).vi"("error in (no error)"=w593, "Message"="Start Sequence", "Message Queue"=w596) -> ("error out"=w595:errorcluster)  [unwired: 1 in, 7 out]
      }
      frame "Instrument Sequence - Stop Sequence" {
        n261 = Unbundle By Name(w602) -> ("Instrument Sequence"=w601:refnum<queue>)
        n262 = call "Enqueue Message (Single).vi"("error in (no error)"=w598, "Message"="Measure Sequence", "Message Queue"=w601) -> ("error out"=w600:errorcluster)  [unwired: 1 in, 7 out]
      }
      frame "Instrument Sequence - Pause Sequence" {
        n263 = Unbundle By Name(w607) -> ("Instrument Sequence"=w606:refnum<queue>)
        n264 = call "Enqueue Message (Single).vi"("error in (no error)"=w603, "Message"="Pause Sequence", "Message Queue"=w606) -> ("error out"=w605:errorcluster)  [unwired: 1 in, 7 out]
      }
      frame "----- StrainElectrical Measurement Events -----" {
        # "NEW DEVICE EVENTS"
      }
      frame "Strain Measurement - Update Strain Sequence" {
        w609 = T58 {"Stress Sequence "={"Max Motor Position"=1380.0, "# Intermediate Points"=5000, "Initial Direction"=enum."Tension"}, "Track?"=FALSE} ("Strain Measurement")
        n265 = Unbundle By Name(w609) -> ("Stress Sequence"=w610:T69)
        n266 = Variant To Data(error in=w619, type=w610, Variant=w618) -> (data=w612:T69, error out=w617:errorcluster)
        n267 = Bundle By Name(cluster=w609, "Stress Sequence"=w612) -> (w611:T58)
        n268 = Unbundle By Name(w613) -> ("Strain Measurement"=w614:refnum<queue>)
        n269 = call "Enqueue Message (Single).vi"("error in (no error)"=w617, "Message Data"=w611, "Message"="Define Strain Sequence", "Message Queue"=w614) -> ("error out"=w616:errorcluster)  [unwired: 7 out]
      }
      frame "Strain Measurement - Start" {
        n270 = Unbundle By Name(w620) -> ("Strain Measurement"=w621:refnum<queue>)
        n271 = call "Enqueue Message (Single).vi"("error in (no error)"=w624, "Message"="Start Strain Measurement", "Message Queue"=w621) -> ("error out"=w623:errorcluster)  [unwired: 1 in, 7 out]
      }
      frame "Strain Measurement - Pause" {
        n272 = Unbundle By Name(w625) -> ("Strain Measurement"=w626:refnum<queue>)
        n273 = call "Enqueue Message (Single).vi"("error in (no error)"=w629, "Message"="Pause", "Message Queue"=w626) -> ("error out"=w628:errorcluster)  [unwired: 1 in, 7 out]
      }
      frame "Strain Measurement - Stop" {
        n274 = Unbundle By Name(w630) -> ("Strain Measurement"=w631:refnum<queue>)
        n275 = call "Enqueue Message (Single).vi"("error in (no error)"=w634, "Message"="Stop", "Message Queue"=w631) -> ("error out"=w633:errorcluster)  [unwired: 1 in, 7 out]
      }
      frame "Strain Measurement - New Sequence" {
        n276 = Unbundle By Name(w639) -> ("Strain Measurement"=w638:refnum<queue>)
        n277 = call "Enqueue Message (Single).vi"("error in (no error)"=w637, "Message"="Clear Instrument Sequence", "Message Queue"=w638) -> ("error out"=w636:errorcluster)  [unwired: 1 in, 7 out]
      }
      frame "Strain Measurement - Add Step" {
        n278 = Unbundle By Name(w644) -> ("Strain Measurement"=w643:refnum<queue>)
        n279 = call "Enqueue Message (Single).vi"("error in (no error)"=w642, "Message"="Add Instrument Sequence Step", "Message Queue"=w643) -> ("error out"=w641:errorcluster)  [unwired: 1 in, 7 out]
      }
      frame "Strain Measurement - Delete Step" {
        n280 = Unbundle By Name(w649) -> ("Strain Measurement"=w648:refnum<queue>)
        n281 = call "Enqueue Message (Single).vi"("error in (no error)"=w647, "Message"="Delete Instrument Sequence Step", "Message Queue"=w648) -> ("error out"=w646:errorcluster)  [unwired: 1 in, 7 out]
      }
      frame "Strain Measurement - Save Sequence" {
        n282 = Unbundle By Name(w654) -> ("Strain Measurement"=w653:refnum<queue>)
        n283 = call "Enqueue Message (Single).vi"("error in (no error)"=w652, "Message"="Save Instrument Sequence", "Message Queue"=w653) -> ("error out"=w651:errorcluster)  [unwired: 1 in, 7 out]
      }
      frame "Strain Measurement - Load Sequence" {
        n284 = Unbundle By Name(w659) -> ("Strain Measurement"=w658:refnum<queue>)
        n285 = call "Enqueue Message (Single).vi"("error in (no error)"=w657, "Message"="Load Instrument Sequence", "Message Queue"=w658) -> ("error out"=w656:errorcluster)  [unwired: 1 in, 7 out]
      }
      frame "----- PlotData Events -----" {
        # "NEW DEVICE EVENTS"
      }
      frame "PlotData - Update Plots" {
        n286 = Variant To Data(error in=w673, type=T62 {"PlotData - Instrument Sequence"=0, "PlotData - Strain Sequence"=0} ("output cluster"), Variant=w672) -> (data=w664:T62, error out=w669:errorcluster)
        n287 = Unbundle By Name(w664) -> ("PlotData - Strain Sequence"=w663:i32, "PlotData - Instrument Sequence"=w662:i32)
        n288 = Bundle By Name(cluster=T51 {"Sliders"={"Strain Sequence"=0, "Instrument Sequence"=0}, "Measurement"={"Which Instrument?"=enum."No Plot", "Electrical Measurement"={"Sequence"=[], "V1"=[], "V2"=[], "V3"=[], "V4"=[], "I1"=[], "I2"=[], "I3"=[], "I4"=[]}, "Measurement Mode"=enum."Sweeping Mode", "Optical Spectrum"={"Intensity"=[], "Wavelength"=[], "Energy"=[], "Raman Shift"=[], "Detector Temperature"=0.0}}, "Instrument Steps"=[], "Strain Points"=[]} ("PlotData Configuration"), "Sliders.Strain Sequence"=w663, "Sliders.Instrument Sequence"=w662) -> (w666:T51)
        n289 = Unbundle By Name(w667) -> ("Plot Data"=w670:refnum<queue>)
        n290 = call "Enqueue Message (Single).vi"("error in (no error)"=w669, "Message Data"=w666, "Message"="Plot Data", "Message Queue"=w670) -> ("error out"=w668:errorcluster)  [unwired: 7 out]
      }
      frame "----- Save Data Events -----" {
        # "Save Data Events"
      }
    }
    n291 = call "Message Handling Loop.vi"("error in (no error)"=w35, "Message Queue"=w33) -> ("dup error in"=w34:errorcluster)  [unwired: 9 out]
  }
  n292 = while "Event Handling Loop" {
    tunnel: w21 -> [w681]
    tunnel: [w680] -> w20
    tunnel: w19 -> [w678]
    tunnel: [w676] -> w18
    stop <- w675 stop-if-true
    n293 = event shown="[3] <user event>: User Event" {
      selector: w681 -> [_ _ _ _ _ _ _ _]
      dyn-events: [_ _ _ _ _ _ _ _] -> w676
      timeout: _ -> [_ _ _ _ _ _ _ _]
      tunnel: [w683 _ w691 _ w698 w705 w707 _] -> w679
      tunnel: w678 -> [w686 w688 w693 w694 w700 w703 w709 w710]
      tunnel: [w682 w688 w692 w694 w699 w704 w708 w710] -> w677
      tunnel: [_ _ _ TRUE ("Priority Message? (F)") _ _ _ _] -> w675
      event Panel Close? {
        # "Send the \"Confirm Quit\" message if the user closes the panel of the VI. Discard the event so the \"Confirm Quit\" message has a chance to run."
        n294 = event-data() -> ()  [unwired: 2 out]
        n295 = call "Enqueue Message (Single).vi"("Priority Message? (F)"=TRUE, "Message"="Initiate Exit", "Message Queue"=w686) -> ("error out"=w683:errorcluster, "dup Message Queue"=w682:refnum<queue>)  [unwired: 2 in, 5 out]
        n296 = event-data("Discard?"=TRUE) -> ()  [unwired: 1 in, 1 out]
      }
      event Application Instance Close {
        # "#CodeRecommended - When a project closes, all VIs within that project are aborted and leave memory. However, any code placed in this event frame is guaranteed to run to completion, so add any cleanup code that absolutely must happen here."
        n297 = event-data() -> ()  [unwired: 2 out]
      }
      event "Exit": Value Change {
        n298 = event-data() -> ()  [unwired: 2 out]
        n299 = call "Enqueue Message (Single).vi"("Priority Message? (F)"=TRUE, "Message"="Initiate Exit", "Message Queue"=w693) -> ("error out"=w691:errorcluster, "dup Message Queue"=w692:refnum<queue>)  [unwired: 2 in, 5 out]
      }
      event User Event {
        n300 = event-data() -> ()  [unwired: 2 out]
      }
      event "Mechanism Motion": Value Change {
        n301 = event-data() -> ()  [unwired: 2 out]
        n302 = call "Enqueue Message (Single).vi"("Message Data"="Mechanism Motion", "Message"="Stress Control - Update Motion Mode", "Message Queue"=w700) -> ("error out"=w698:errorcluster, "dup Message Queue"=w699:refnum<queue>)  [unwired: 1 in, 6 out]
      }
      event "Destination (°)": Value Change {
        n303 = event-data() -> ()  [unwired: 2 out]
        n304 = call "Enqueue Message (Single).vi"("Message Data"="Destination (°)", "Message"="Stress Control - Update Destination", "Message Queue"=w703) -> ("error out"=w705:errorcluster, "dup Message Queue"=w704:refnum<queue>)  [unwired: 1 in, 6 out]
      }
      event "Apply Stress": Value Change {
        n305 = event-data() -> ()  [unwired: 2 out]
        n306 = call "Enqueue Message (Single).vi"("Message"="Stress Control - Change Stress", "Message Queue"=w709) -> ("error out"=w707:errorcluster, "dup Message Queue"=w708:refnum<queue>)  [unwired: 2 in, 6 out]
      }
      event "Stop": Value Change {
        n307 = event-data() -> ()  [unwired: 2 out]
      }
    }
    n308 = call "Event Handling Loop.vi"("error in (no error)"=w679, "Message Queue"=w677) -> ("dup error in"=w680:errorcluster)  [unwired: 9 out]
  }
  n309 = Unregister For Events(event registration refnum=w18, error in=w20) -> (error out=w5:errorcluster)
  n310 = Merge Errors(w5, w4, w3) -> (w13:errorcluster)
  n311 = call "Close Notifiers.vi"("error in"=w13, "Notifiers"=w6) -> ("error out"=w12:errorcluster)  [unwired: 9 out]
  n312 = call "Destroy User Event - Stop.vi"("error in (no error)"=w12, "User Event - Stop"=w14) -> ("error out"=w17:errorcluster)  [unwired: 9 out]
  n313 = property class="App"(error in=w17) -> (error out=w15:errorcluster, "App.Kind"=w16:T70)  [unwired: 1 in, 1 out]
  n314 = case shown="\"Development System\"" w16 {
    tunnel: w15 -> [w711 w712 _ _ _ _ _]
    frame "invalid app kind", Default {
      n315 = call <vilib>:"Simple Error Handler.vi"("error in (no error)"=w711) -> ()  [unwired: 1 in, 8 out]
    }
    frame "Development System" {
      n316 = call <vilib>:"Simple Error Handler.vi"("error in (no error)"=w712) -> ()  [unwired: 1 in, 8 out]
    }
    frame "Run Time System" {
      n317 = Quit LabVIEW() -> ()  [unwired: 1 out]
    }
    frame "Student Edition" {
    }
    frame "Embedded LabVIEW" {
    }
    frame "Evaluation" {
    }
    frame "Custom" {
    }
  }
